vi "GameController.vi"() -> ()   [LabVIEW 2026]
uses:
  <vilib>/Utility/config.llb/Read Key (String).vi
  Instance          15 22Saved   GameController .vi
  <vilib>/Utility/config.llb/Write Key (String).vi
  <vilib>/Instr/_visa.llb/VISA Configure Serial Port (Instr).vi
  <vilib>/Utility/config.llb/NI_LVConfig.lvlib
panel:
  out "Team / Player":string
  out "COM Port":bool
  out "Communication":bool
  in  "Tab Control":T1(tab)
  in  "Final Jeopardy Time":u8=30
  out "Used 7":string
  in  "Final Jeopardy":path
  in  "Question Time":u8=10
  in  "Answer Time":u8=5
  in  "Initialize Moderator Module":bool
  in  "COM Port":refnum<visa-resource-name>
  in  "Point Multiplier":u16(ring) items=["Normal Points", "Double Points"]
  in  "Wrong Sound":path=path "C:/Program Files/BetaBowl/Controller/WrongSound.wav"
  in  "Right Sound":path=path "C:/Program Files/BetaBowl/Controller/RightSound.wav"
  out "Used 6":string
  out "Used 5":string
  out "Used 4":string
  out "Used 3":string
  out "Used 2":string
  out "Used 1":string
  in  "Start Game":bool
  in  "Question Setting":u16(ring) items=["Play & Display Questions", "Display Questions Only"]
  in  "Teams":u16(ring) items=["Two Teams", "Three Teams"]
  in  "Category 6":path
  in  "Category 5":path
  in  "Category 4":path
  in  "Category 3":path
  in  "Category 2":path
  in  "Category 1":path
  in  "Final Jeopardy":bool
  out "GameGUI":bool[][](array[boolean])
  in  "Play/Display Question":bool
  out "Answer":string
  out "Question":string
  in  "TEAM 3":string="0"
  in  "TEAM 2":string="0"
  in  "TEAM 1":string="0"
  in  "WRONG":bool
  in  "RIGHT":bool
  in  "Play/Display":bool
  out "Special Answer":string
  out "Special Question":string
  in  "Team 3 W/R?":bool
  in  "Team 2 W/R?":bool
  in  "Team 1 W/R?":bool
  in  "Dialog Done":bool
  in  "WAGER TEAM 3":string="0"
  in  "WAGER TEAM 2":string="0"
  in  "WAGER TEAM 1":string="0"
  out "Received Message":string
  out "Stats":i32[](array[numeric])
  out "Is Daily Double or Final Jeopardy":bool
  out "Game Started":bool
  out "Timeout":bool
  in  "Start New Question":bool
  out "Com Msgs":string
  out "Daily Double Questions":i32[](array[numeric])
  out "Daily Double Categories":i32[](array[numeric])
  in  "Button Pressed":i32
  in  "Team Pressed":i32
  out "Question":u8
  out "Category":u8
  in  "stop":bool
  # "Category"
  # "Last Used"
  # "1"
  # "2"
  # "3"
  # "4"
  # "5"
  # "6"
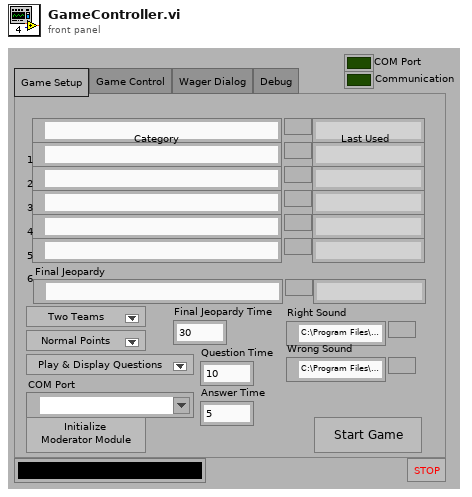
[diagram p1: front panel]
types:
  T1 = enum32{"Game Setup", "Game Control", "Wager Dialog", "Debug"}
  T2 = enum32{"Game Setup", "Game Control", "Wager Dialog"}
  T3 = typedef "NI_LVConfig.lvlib/Config Data RefNum.ctl" = refnum<k1>
  T4 = typedef "Sound Format.ctl" = cluster{"sound quality":enum16{"mono", "stereo"}, "rate":enum16{"11025", "22050", "44100", "8000"}, "bits per sample":enum16{"8 bit", "16 bit"}}
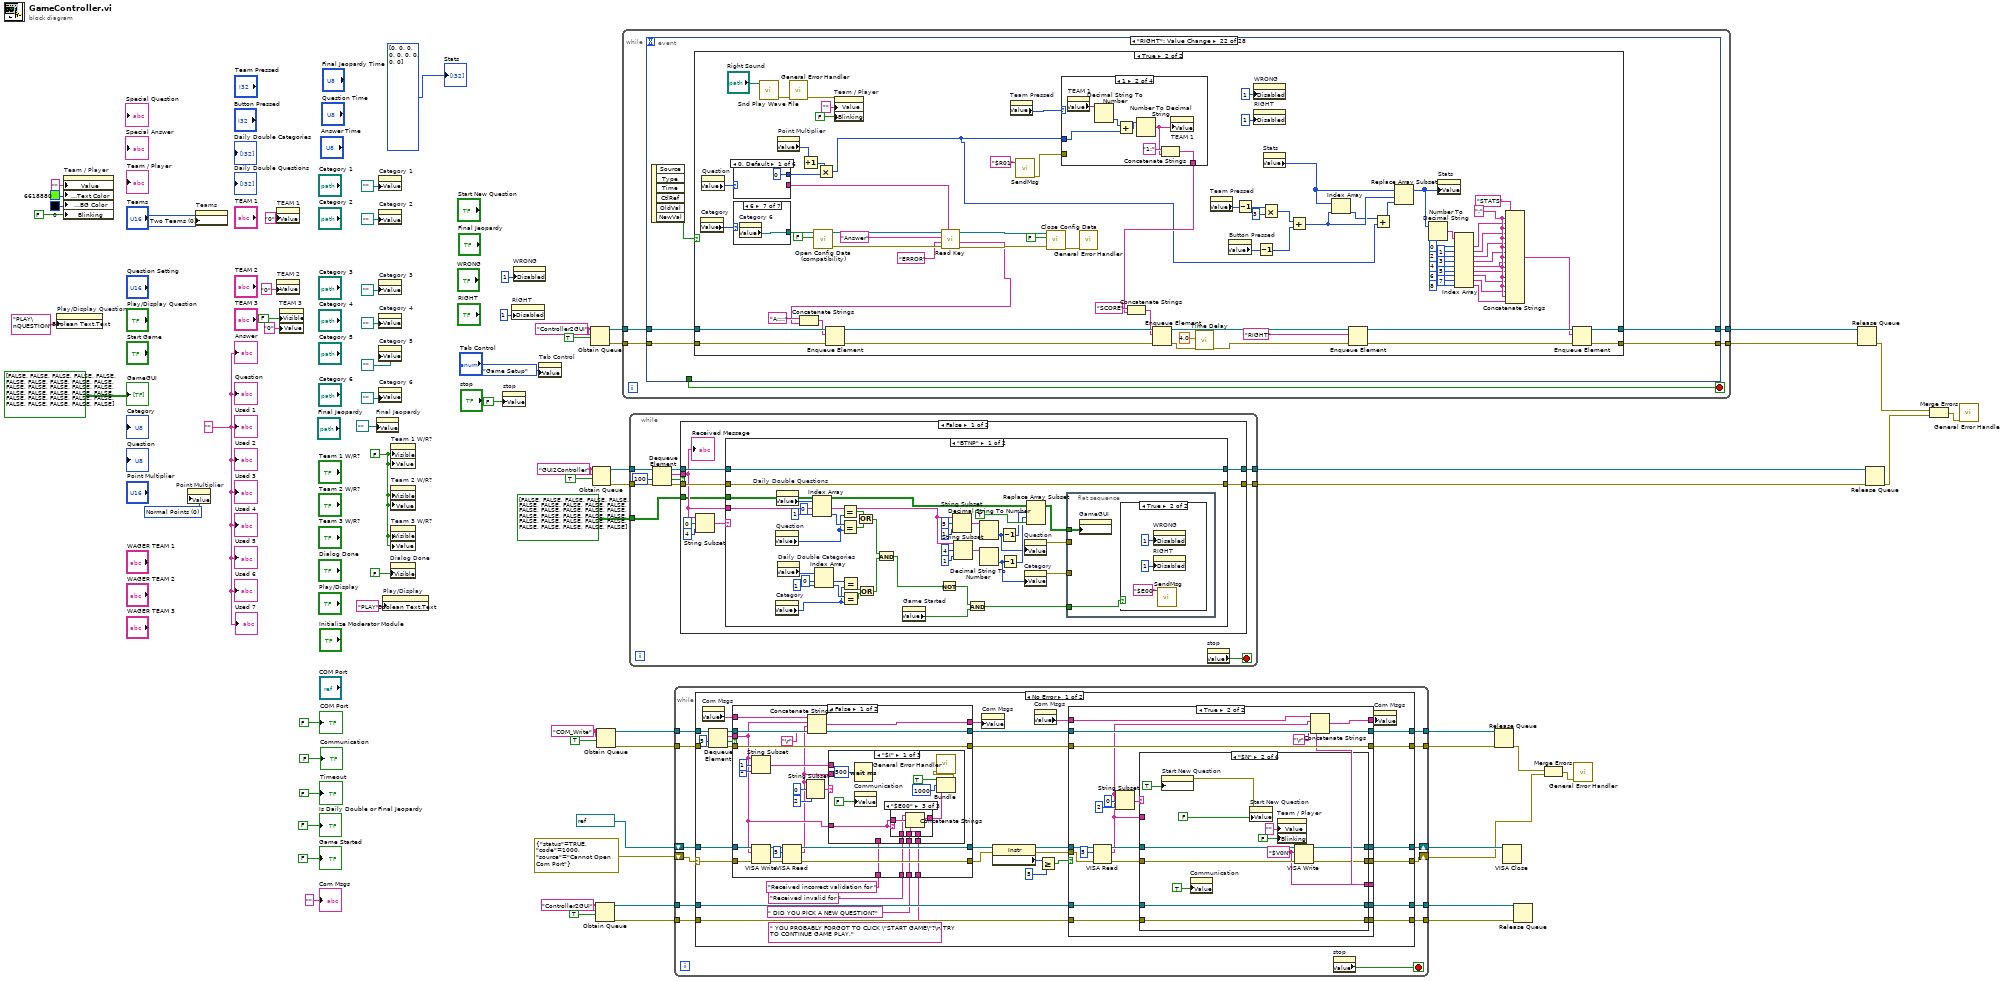
[diagram p0: block diagram]
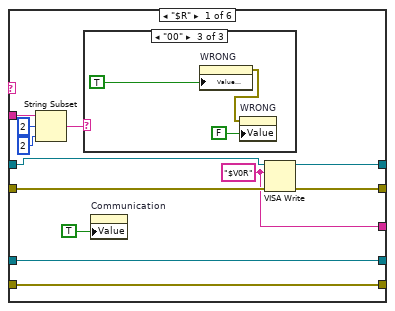
[diagram p3: hidden frame]
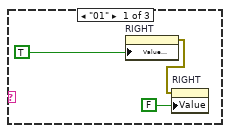
[diagram p4: hidden frame]
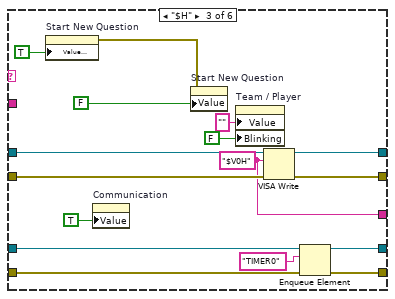
[diagram p6: hidden frame]
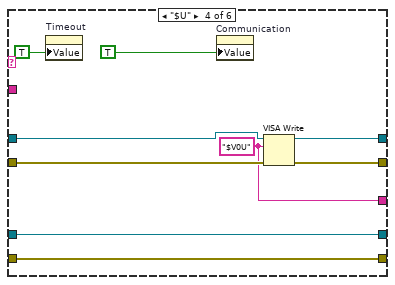
[diagram p7: hidden frame]
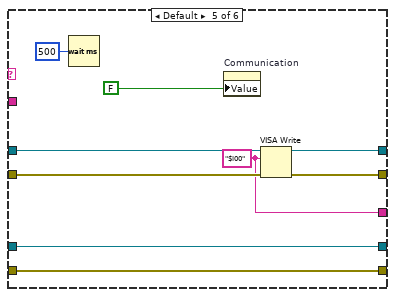
[diagram p8: hidden frame]
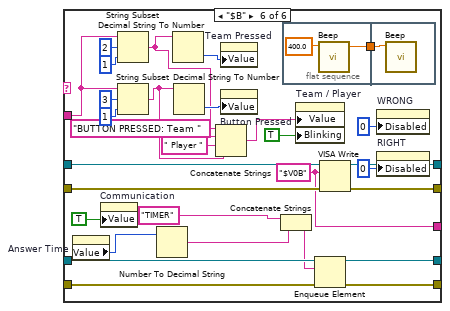
[diagram p9: hidden frame]
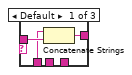
[diagram p10: hidden frame]
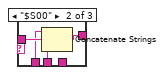
[diagram p11: hidden frame]
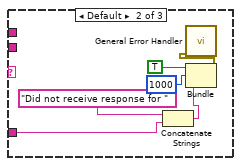
[diagram p12: hidden frame]
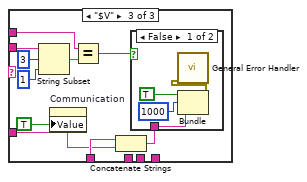
[diagram p13: hidden frame]
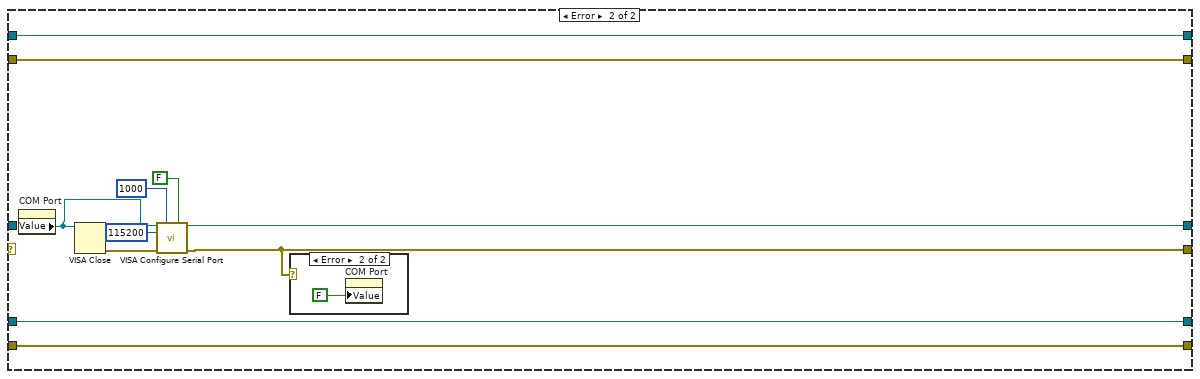
[diagram p16: hidden frame]
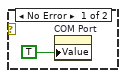
[diagram p17: hidden frame]
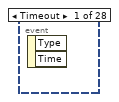
[diagram p18: hidden frame]
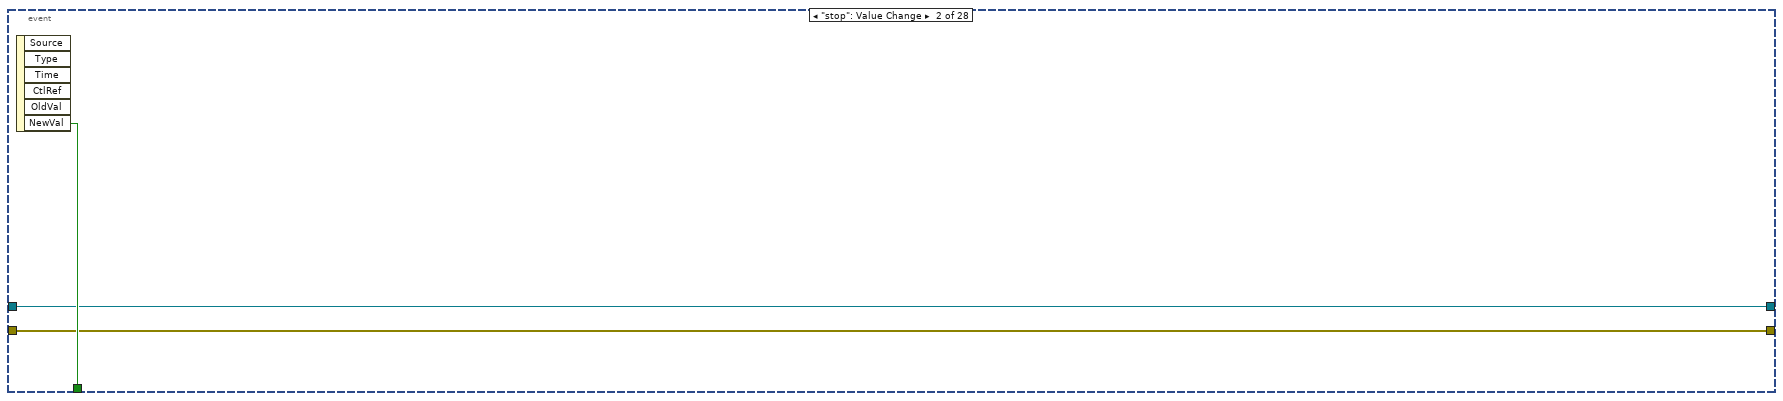
[diagram p19: hidden frame]
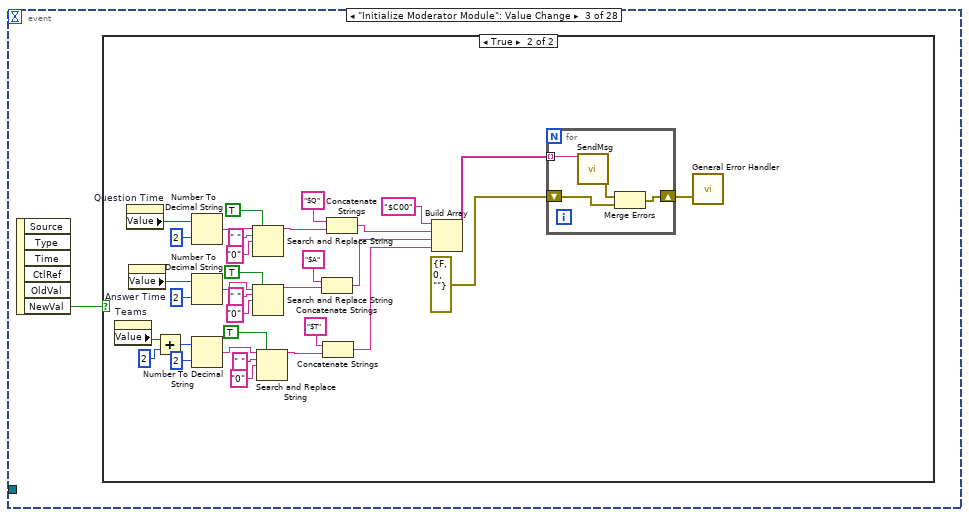
[diagram p20: hidden frame]
diagram:
  w17 = "Controller2GUI" ("name (unnamed)")
  w31 = "COM_Write" ("name (unnamed)")
  w34 = u16 0 items=["Normal Points", "Double Points"] ("Point Multiplier")
  w38 = FALSE ("Visible")
  w4 = "" ("Modified 1")
  w47 = u16 0 items=["Two Teams", "Three Teams"] ("Teams")
  w61 = "Controller2GUI" ("name (unnamed)")
  w68 = "GUI2Controller" ("name (unnamed)")
  n1 = property on="Play/Display Question" class="Bool (strict)"("Boolean Text.Text"="PLAY\nQUESTION") -> ()  [unwired: 2 in, 2 out]
  n2 = property on="Team / Player" class="Str"("Value"="" ("Team / Player"), "Text.Text Colors:Text Color"=u32 6618880, "Text.Text Colors:BG Color"=u32 0, "Blinking"=FALSE) -> ()  [unwired: 2 in, 2 out]
  n3 = property on="Point Multiplier" class="Ring (strict)"("Value"=w34) -> ()  [unwired: 2 in, 2 out]
  n4 = property on="Teams" class="Ring (strict)"("Value (Signaling)"=w47) -> ()  [unwired: 2 in, 2 out]
  n5 = property on="TEAM 1" class="Str"("Value"="0" ("TEAM 1")) -> ()  [unwired: 2 in, 2 out]
  n6 = property on="TEAM 2" class="Str"("Value"="0" ("TEAM 2")) -> ()  [unwired: 2 in, 2 out]
  n7 = property on="TEAM 3" class="Str"("Visible"=FALSE, "Value"="0" ("TEAM 3")) -> ()  [unwired: 2 in, 2 out]
  n8 = property on="Final Jeopardy" class="Path"("Value"=path "" ("Final Jeopardy")) -> ()  [unwired: 2 in, 2 out]
  n9 = property on="Category 1" class="Path"("Value"=path "" ("Category 1")) -> ()  [unwired: 2 in, 2 out]
  n10 = property on="Category 2" class="Path"("Value"=path "" ("Category 2")) -> ()  [unwired: 2 in, 2 out]
  n11 = property on="Category 3" class="Path"("Value"=path "" ("Category 3")) -> ()  [unwired: 2 in, 2 out]
  n12 = property on="Category 4" class="Path"("Value"=path "" ("Category 4")) -> ()  [unwired: 2 in, 2 out]
  n13 = property on="Category 5" class="Path"("Value"=path "" ("Category 5")) -> ()  [unwired: 2 in, 2 out]
  n14 = property on="Category 6" class="Path"("Value"=path "" ("Category 6")) -> ()  [unwired: 2 in, 2 out]
  n15 = property on="Play/Display" class="Bool (strict)"("Boolean Text.Text"="PLAY") -> ()  [unwired: 2 in, 2 out]
  n16 = property on="Dialog Done" class="Bool (strict)"("Visible"=FALSE) -> ()  [unwired: 2 in, 2 out]
  n17 = property on="Team 1 W/R?" class="Bool (strict)"("Visible"=w38, "Value"=w38) -> ()  [unwired: 2 in, 2 out]
  n18 = property on="Team 2 W/R?" class="Bool (strict)"("Visible"=w38, "Value"=w38) -> ()  [unwired: 2 in, 2 out]
  n19 = property on="Team 3 W/R?" class="Bool (strict)"("Visible"=w38, "Value"=w38) -> ()  [unwired: 2 in, 2 out]
  n20 = property on="stop" class="Bool (strict)"("Value"=FALSE ("stop")) -> ()  [unwired: 2 in, 2 out]
  n21 = property on="RIGHT" class="Bool (strict)"("Disabled"=u8 1) -> ()  [unwired: 2 in, 2 out]
  n22 = property on="WRONG" class="Bool (strict)"("Disabled"=u8 1) -> ()  [unwired: 2 in, 2 out]
  n23 = property on="Tab Control" class="TabCtl (strict)"("Value"=T2."Game Setup" ("Tab Control")) -> ()  [unwired: 2 in, 2 out]
  n24 = Obtain Queue(name (unnamed)=w61, element data type=w61, create if not found? (T)=TRUE) -> (queue out=w59:refnum<queue>, error out=w60:errorcluster)  [unwired: 2 in, 1 out]
  n25 = Obtain Queue(name (unnamed)=w68, element data type=w68, create if not found? (T)=TRUE) -> (queue out=w65:refnum<queue>, error out=w66:errorcluster)  [unwired: 2 in, 1 out]
  n26 = Obtain Queue(name (unnamed)=w17, element data type=w17, create if not found? (T)=TRUE) -> (queue out=w15:refnum<queue>, error out=w14:errorcluster)  [unwired: 2 in, 1 out]
  n27 = Obtain Queue(name (unnamed)=w31, element data type=w31, create if not found? (T)=TRUE) -> (queue out=w29:refnum<queue>, error out=w30:errorcluster)  [unwired: 2 in, 1 out]
  n28 = while {
    tunnel: w60 -> [w72]
    tunnel: w59 -> [w71]
    tunnel: [w70] -> w58
    tunnel: [w69] -> w57
    stop <- w73 stop-if-true
    n29 = event shown="[21] \"RIGHT\": Value Change" {
      selector: _ -> [_ _ _ _ _ _ _ _ _ _ _ _ _ _ _ _ _ _ _ _ _ _ _ _ _ _ _ _]
      dyn-events: _ -> [_ _ _ _ _ _ _ _ _ _ _ _ _ _ _ _ _ _ _ _ _ _ _ _ _ _ _ _]
      timeout: _ -> [_ _ _ _ _ _ _ _ _ _ _ _ _ _ _ _ _ _ _ _ _ _ _ _ _ _ _ _]
      tunnel: [_ w76 _ _ _ _ _ _ _ _ _ _ _ _ _ _ _ _ _ _ _ _ _ _ _ _ _ _] -> w73
      tunnel: w72 -> [_ w74 _ w128 w152 w175 w198 w221 w244 w253 w273 w291 w298 w305 w310 w317 w324 w330 _ w417 w438 w454 w578 w711 w762 w866 _ w1124]
      tunnel: w71 -> [_ w75 _ w129 w153 w176 w199 w222 w245 w254 w274 w292 w299 w306 w311 w318 w325 w331 _ w418 w439 w455 w579 w712 w763 w867 _ w1125]
      tunnel: [_ w75 _ w127 w151 w174 w197 w220 w243 w254 w272 w287 w294 w301 w308 w315 w322 w329 _ w416 w437 w453 w577 w710 w761 w865 _ w1123] -> w70
      tunnel: [_ w74 _ w126 w150 w173 w196 w219 w242 w253 w271 w286 w293 w300 w307 w314 w321 w328 _ w415 w436 w452 w576 w709 w760 w864 _ w1122] -> w69
      event Timeout {
        n30 = event-data() -> ()  [unwired: 1 in, 2 out]
      }
      event "stop": Value Change {
        n31 = event-data() -> ("NewVal"=w76:bool)  [unwired: 1 in, 5 out]
      }
      event "Initialize Moderator Module": Value Change {
        n32 = event-data() -> ("NewVal"=w77:bool)  [unwired: 1 in, 5 out]
        n33 = case shown="True" w77 {
          frame False {
          }
          frame True {
            n34 = property on="Teams" class="Ring (strict)"() -> ("Value"=w79:u16)  [unwired: 2 in, 2 out]
            n35 = property on="Question Time" class="DigNum (strict)"() -> ("Value"=w106:u8)  [unwired: 2 in, 2 out]
            n36 = property on="Answer Time" class="DigNum (strict)"() -> ("Value"=w107:u8)  [unwired: 2 in, 2 out]
            n37 = Add(x=w79, y=u16 2) -> (x+y=w80:u16)
            n38 = Number To Decimal String(number=w106, width (-)=i16 2) -> (decimal integer string=w95:string)
            n39 = Number To Decimal String(number=w107, width (-)=i16 2) -> (decimal integer string=w84:string)
            n40 = Number To Decimal String(number=w80, width (-)=i16 2) -> (decimal integer string=w82:string)
            n41 = Search and Replace String(replace all?=TRUE ("replace all? (F)"), input string=w95, search string=" ", replace string="0" ("replace string (\"\")")) -> (result string=w94:string)  [unwired: 4 in, 3 out]
            n42 = Search and Replace String(replace all?=TRUE ("replace all? (F)"), input string=w84, search string=" ", replace string="0" ("replace string (\"\")")) -> (result string=w83:string)  [unwired: 4 in, 3 out]
            n43 = Search and Replace String(replace all?=TRUE ("replace all? (F)"), input string=w82, search string=" ", replace string="0" ("replace string (\"\")")) -> (result string=w81:string)  [unwired: 4 in, 3 out]
            n44 = Concatenate Strings("$A", w83) -> (w100:string)
            n45 = Concatenate Strings("$T", w81) -> (w97:string)
            n46 = Concatenate Strings("$Q", w94) -> (w102:string)
            n47 = Build Array("$C00", w102, w100, w97) -> (w109:string[])
            n48 = for {
              shift-right: [w112] -> w96
              shift-left: errorcluster {"status"=FALSE, "code"=0, "source"=""} ("error in (no error)") -> [w113]
              tunnel: w109 -> [w111] mode=indexing
              n49 = call "SendMsg.vi"("Data"=w111) -> ("error out"=w114:errorcluster)  [unwired: 14 in]
              n50 = Merge Errors(w114, w113) -> (w112:errorcluster)
            }
            n51 = call <vilib>:"General Error Handler.vi"("error in (no error)"=w96) -> ()  [unwired: 10 in, 5 out]
          }
        }
      }
      event "Category 1": Value Change {
        n52 = event-data() -> ("NewVal"=w137:path)  [unwired: 1 in, 5 out]
        n53 = call <vilib>:"Open Config Data (compatibility).vi"("create file if necessary (T)"=FALSE ("create file if necessary? (T)"), "configuration file path"=w137) -> ("error out"=w134:errorcluster, "refnum"=w135:T3)  [unwired: 7 in, 1 out]
        n54 = call-poly <vilib>:"Read Key.vi"("section"="HEADER", "error in (no error)"=w134, "default value"="ERROR" ("key"), "key"="CategoryName", "refnum"=w135) -> ("error out"=w120:errorcluster, "value"=w123:string, "refnum out"=w122:T3)  [unwired: 3 in, 1 out]
        n55 = Concatenate Strings("CAT1:" ("string"), w123) -> (w125:string)
        n56 = call-poly <vilib>:"Read Key.vi"("section"="HEADER", "error in (no error)"=w120, "default value"="ERROR" ("key"), "key"="Used", "refnum"=w122) -> ("error out"=w119:errorcluster, "value"=w115:string, "refnum out"=w121:T3)  [unwired: 3 in, 1 out]
        n57 = property on="Used 1" class="Str"("Value"=w115) -> ()  [unwired: 2 in, 2 out]
        n58 = Enqueue Element(queue=w129, element=w125, error in (no error)=w128) -> (queue out=w127:refnum<queue>, error out=w126:errorcluster)  [unwired: 1 in, 1 out]
        n59 = call <vilib>:"Close Config Data.vi"("error in (no error)"=w119, "write file if changed (T)"=FALSE ("write configuration file? (T)"), "refnum"=w121) -> ()  [unwired: 7 in, 2 out]
      }
      event "Category 2": Value Change {
        n60 = event-data() -> ("NewVal"=w160:path)  [unwired: 1 in, 5 out]
        n61 = call <vilib>:"Open Config Data (compatibility).vi"("create file if necessary (T)"=FALSE ("create file if necessary? (T)"), "configuration file path"=w160) -> ("error out"=w157:errorcluster, "refnum"=w158:T3)  [unwired: 7 in, 1 out]
        n62 = call-poly <vilib>:"Read Key.vi"("section"="HEADER", "error in (no error)"=w157, "default value"="ERROR" ("key"), "key"="CategoryName", "refnum"=w158) -> ("error out"=w139:errorcluster, "value"=w147:string, "refnum out"=w140:T3)  [unwired: 3 in, 1 out]
        n63 = Concatenate Strings("CAT2:" ("string"), w147) -> (w149:string)
        n64 = call-poly <vilib>:"Read Key.vi"("section"="HEADER", "error in (no error)"=w139, "default value"="ERROR" ("key"), "key"="Used", "refnum"=w140) -> ("error out"=w144:errorcluster, "value"=w138:string, "refnum out"=w145:T3)  [unwired: 3 in, 1 out]
        n65 = property on="Used 2" class="Str"("Value"=w138) -> ()  [unwired: 2 in, 2 out]
        n66 = Enqueue Element(queue=w153, element=w149, error in (no error)=w152) -> (queue out=w151:refnum<queue>, error out=w150:errorcluster)  [unwired: 1 in, 1 out]
        n67 = call <vilib>:"Close Config Data.vi"("error in (no error)"=w144, "write file if changed (T)"=FALSE ("write configuration file? (T)"), "refnum"=w145) -> ()  [unwired: 7 in, 2 out]
      }
      event "Category 3": Value Change {
        n68 = event-data() -> ("NewVal"=w183:path)  [unwired: 1 in, 5 out]
        n69 = call <vilib>:"Open Config Data (compatibility).vi"("create file if necessary (T)"=FALSE ("create file if necessary? (T)"), "configuration file path"=w183) -> ("error out"=w180:errorcluster, "refnum"=w181:T3)  [unwired: 7 in, 1 out]
        n70 = call-poly <vilib>:"Read Key.vi"("section"="HEADER", "error in (no error)"=w180, "default value"="ERROR" ("key"), "key"="CategoryName", "refnum"=w181) -> ("error out"=w162:errorcluster, "value"=w170:string, "refnum out"=w163:T3)  [unwired: 3 in, 1 out]
        n71 = Concatenate Strings("CAT3:" ("string"), w170) -> (w172:string)
        n72 = call-poly <vilib>:"Read Key.vi"("section"="HEADER", "error in (no error)"=w162, "default value"="ERROR" ("key"), "key"="Used", "refnum"=w163) -> ("error out"=w166:errorcluster, "value"=w161:string, "refnum out"=w167:T3)  [unwired: 3 in, 1 out]
        n73 = Enqueue Element(queue=w176, element=w172, error in (no error)=w175) -> (queue out=w174:refnum<queue>, error out=w173:errorcluster)  [unwired: 1 in, 1 out]
        n74 = property on="Used 3" class="Str"("Value"=w161) -> ()  [unwired: 2 in, 2 out]
        n75 = call <vilib>:"Close Config Data.vi"("error in (no error)"=w166, "write file if changed (T)"=FALSE ("write configuration file? (T)"), "refnum"=w167) -> ()  [unwired: 7 in, 2 out]
      }
      event "Category 4": Value Change {
        n76 = event-data() -> ("NewVal"=w206:path)  [unwired: 1 in, 5 out]
        n77 = call <vilib>:"Open Config Data (compatibility).vi"("create file if necessary (T)"=FALSE ("create file if necessary? (T)"), "configuration file path"=w206) -> ("error out"=w203:errorcluster, "refnum"=w204:T3)  [unwired: 7 in, 1 out]
        n78 = call-poly <vilib>:"Read Key.vi"("section"="HEADER", "error in (no error)"=w203, "default value"="ERROR" ("key"), "key"="CategoryName", "refnum"=w204) -> ("error out"=w185:errorcluster, "value"=w193:string, "refnum out"=w186:T3)  [unwired: 3 in, 1 out]
        n79 = Concatenate Strings("CAT4:" ("string"), w193) -> (w195:string)
        n80 = call-poly <vilib>:"Read Key.vi"("section"="HEADER", "error in (no error)"=w185, "default value"="ERROR" ("key"), "key"="Used", "refnum"=w186) -> ("error out"=w189:errorcluster, "value"=w184:string, "refnum out"=w190:T3)  [unwired: 3 in, 1 out]
        n81 = Enqueue Element(queue=w199, element=w195, error in (no error)=w198) -> (queue out=w197:refnum<queue>, error out=w196:errorcluster)  [unwired: 1 in, 1 out]
        n82 = property on="Used 4" class="Str"("Value"=w184) -> ()  [unwired: 2 in, 2 out]
        n83 = call <vilib>:"Close Config Data.vi"("error in (no error)"=w189, "write file if changed (T)"=FALSE ("write configuration file? (T)"), "refnum"=w190) -> ()  [unwired: 7 in, 2 out]
      }
      event "Category 5": Value Change {
        n84 = event-data() -> ("NewVal"=w229:path)  [unwired: 1 in, 5 out]
        n85 = call <vilib>:"Open Config Data (compatibility).vi"("create file if necessary (T)"=FALSE ("create file if necessary? (T)"), "configuration file path"=w229) -> ("error out"=w226:errorcluster, "refnum"=w227:T3)  [unwired: 7 in, 1 out]
        n86 = call-poly <vilib>:"Read Key.vi"("section"="HEADER", "error in (no error)"=w226, "default value"="ERROR" ("key"), "key"="CategoryName", "refnum"=w227) -> ("error out"=w208:errorcluster, "value"=w216:string, "refnum out"=w209:T3)  [unwired: 3 in, 1 out]
        n87 = Concatenate Strings("CAT5:" ("string"), w216) -> (w218:string)
        n88 = call-poly <vilib>:"Read Key.vi"("section"="HEADER", "error in (no error)"=w208, "default value"="ERROR" ("key"), "key"="Used", "refnum"=w209) -> ("error out"=w212:errorcluster, "value"=w207:string, "refnum out"=w213:T3)  [unwired: 3 in, 1 out]
        n89 = Enqueue Element(queue=w222, element=w218, error in (no error)=w221) -> (queue out=w220:refnum<queue>, error out=w219:errorcluster)  [unwired: 1 in, 1 out]
        n90 = property on="Used 5" class="Str"("Value"=w207) -> ()  [unwired: 2 in, 2 out]
        n91 = call <vilib>:"Close Config Data.vi"("error in (no error)"=w212, "write file if changed (T)"=FALSE ("write configuration file? (T)"), "refnum"=w213) -> ()  [unwired: 7 in, 2 out]
      }
      event "Category 6": Value Change {
        n92 = event-data() -> ("NewVal"=w252:path)  [unwired: 1 in, 5 out]
        n93 = call <vilib>:"Open Config Data (compatibility).vi"("create file if necessary (T)"=FALSE ("create file if necessary? (T)"), "configuration file path"=w252) -> ("error out"=w249:errorcluster, "refnum"=w250:T3)  [unwired: 7 in, 1 out]
        n94 = call-poly <vilib>:"Read Key.vi"("section"="HEADER", "error in (no error)"=w249, "default value"="ERROR" ("key"), "key"="CategoryName", "refnum"=w250) -> ("error out"=w231:errorcluster, "value"=w239:string, "refnum out"=w232:T3)  [unwired: 3 in, 1 out]
        n95 = Concatenate Strings("CAT6:" ("string"), w239) -> (w241:string)
        n96 = call-poly <vilib>:"Read Key.vi"("section"="HEADER", "error in (no error)"=w231, "default value"="ERROR" ("key"), "key"="Used", "refnum"=w232) -> ("error out"=w235:errorcluster, "value"=w230:string, "refnum out"=w236:T3)  [unwired: 3 in, 1 out]
        n97 = Enqueue Element(queue=w245, element=w241, error in (no error)=w244) -> (queue out=w243:refnum<queue>, error out=w242:errorcluster)  [unwired: 1 in, 1 out]
        n98 = property on="Used 6" class="Str"("Value"=w230) -> ()  [unwired: 2 in, 2 out]
        n99 = call <vilib>:"Close Config Data.vi"("error in (no error)"=w235, "write file if changed (T)"=FALSE ("write configuration file? (T)"), "refnum"=w236) -> ()  [unwired: 7 in, 2 out]
      }
      event "Final Jeopardy": Value Change {
        n100 = event-data() -> ("NewVal"=w270:path)  [unwired: 1 in, 5 out]
        n101 = call <vilib>:"Open Config Data (compatibility).vi"("create file if necessary (T)"=FALSE ("create file if necessary? (T)"), "configuration file path"=w270) -> ("error out"=w267:errorcluster, "refnum"=w268:T3)  [unwired: 7 in, 1 out]
        n102 = call-poly <vilib>:"Read Key.vi"("section"="HEADER", "error in (no error)"=w267, "default value"="ERROR" ("key"), "key"="CategoryName", "refnum"=w268) -> ("error out"=w256:errorcluster, "refnum out"=w257:T3)  [unwired: 3 in, 2 out]
        n103 = call-poly <vilib>:"Read Key.vi"("section"="HEADER", "error in (no error)"=w256, "default value"="ERROR" ("key"), "key"="Used", "refnum"=w257) -> ("error out"=w260:errorcluster, "value"=w255:string, "refnum out"=w261:T3)  [unwired: 3 in, 1 out]
        n104 = property on="Used 7" class="Str"("Value"=w255) -> ()  [unwired: 2 in, 2 out]
        n105 = call <vilib>:"Close Config Data.vi"("error in (no error)"=w260, "write file if changed (T)"=FALSE ("write configuration file? (T)"), "refnum"=w261) -> ()  [unwired: 7 in, 2 out]
      }
      event "Start New Question": Value Change {
        n106 = event-data() -> ("NewVal"=w275:bool)  [unwired: 1 in, 5 out]
        n107 = case shown="True" w275 {
          tunnel: w274 -> [w277 w281]
          tunnel: w273 -> [w276 w280]
          tunnel: [w277 w284] -> w272
          tunnel: [w276 w283] -> w271
          frame False {
          }
          frame True {
            n108 = Enqueue Element(queue=w281, element="TAB::BOARD", error in (no error)=w280) -> (queue out=w278:refnum<queue>, error out=w279:errorcluster)  [unwired: 1 in, 1 out]
            n109 = Enqueue Element(queue=w278, element="UNLOC", error in (no error)=w279) -> (queue out=w284:refnum<queue>, error out=w283:errorcluster)  [unwired: 1 in, 1 out]
          }
        }
      }
      event "TEAM 1": Value Change {
        n110 = event-data() -> ("NewVal"=w289:string)  [unwired: 1 in, 5 out]
        n111 = Concatenate Strings("SCORE1:" ("string"), w289) -> (w288:string)
        n112 = Enqueue Element(queue=w292, element=w288, error in (no error)=w291) -> (queue out=w287:refnum<queue>, error out=w286:errorcluster)  [unwired: 1 in, 1 out]
      }
      event "TEAM 2": Value Change {
        n113 = event-data() -> ("NewVal"=w296:string)  [unwired: 1 in, 5 out]
        n114 = Concatenate Strings("SCORE2:" ("string"), w296) -> (w295:string)
        n115 = Enqueue Element(queue=w299, element=w295, error in (no error)=w298) -> (queue out=w294:refnum<queue>, error out=w293:errorcluster)  [unwired: 1 in, 1 out]
      }
      event "TEAM 3": Value Change {
        n116 = event-data() -> ("NewVal"=w303:string)  [unwired: 1 in, 5 out]
        n117 = Concatenate Strings("SCORE3:" ("string"), w303) -> (w302:string)
        n118 = Enqueue Element(queue=w306, element=w302, error in (no error)=w305) -> (queue out=w301:refnum<queue>, error out=w300:errorcluster)  [unwired: 1 in, 1 out]
      }
      event "WAGER TEAM 1": Value Change {
        n119 = event-data() -> ("NewVal"=w309:string)  [unwired: 1 in, 5 out]
        n120 = Concatenate Strings("WT1::" ("string"), w309) -> (w312:string)
        n121 = Enqueue Element(queue=w311, element=w312, error in (no error)=w310) -> (queue out=w308:refnum<queue>, error out=w307:errorcluster)  [unwired: 1 in, 1 out]
      }
      event "WAGER TEAM 2": Value Change {
        n122 = event-data() -> ("NewVal"=w316:string)  [unwired: 1 in, 5 out]
        n123 = Concatenate Strings("WT2::" ("string"), w316) -> (w319:string)
        n124 = Enqueue Element(queue=w318, element=w319, error in (no error)=w317) -> (queue out=w315:refnum<queue>, error out=w314:errorcluster)  [unwired: 1 in, 1 out]
      }
      event "WAGER TEAM 3": Value Change {
        n125 = event-data() -> ("NewVal"=w323:string)  [unwired: 1 in, 5 out]
        n126 = Concatenate Strings("WT3::" ("string"), w323) -> (w326:string)
        n127 = Enqueue Element(queue=w325, element=w326, error in (no error)=w324) -> (queue out=w322:refnum<queue>, error out=w321:errorcluster)  [unwired: 1 in, 1 out]
      }
      event "Dialog Done": Value Change {
        n128 = event-data() -> ("NewVal"=w332:bool)  [unwired: 1 in, 5 out]
        n129 = case shown="True" w332 {
          tunnel: w331 -> [w333 w336]
          tunnel: w330 -> [w334 w335]
          tunnel: [w333 w360] -> w329
          tunnel: [w334 w359] -> w328
          frame False {
          }
          frame True {
            n130 = property on="Tab Control" class="TabCtl (strict)"("Value"=T2."Game Control" ("Tab Control")) -> (error out=w388:errorcluster)  [unwired: 2 in, 1 out]
            n131 = Enqueue Element(queue=w336, element="TIMER0", error in (no error)=w335) -> (queue out=w337:refnum<queue>, error out=w338:errorcluster)  [unwired: 1 in, 1 out]
            n132 = property on="WAGER TEAM 2" class="Str"() -> ("Value"=w367:string)  [unwired: 2 in, 2 out]
            n133 = property on="WAGER TEAM 3" class="Str"() -> ("Value"=w366:string)  [unwired: 2 in, 2 out]
            n134 = property on="WAGER TEAM 1" class="Str"() -> ("Value"=w368:string)  [unwired: 2 in, 2 out]
            n135 = property on="Dialog Done" class="Bool (strict)"(error in=w388, "Visible"=FALSE) -> ()  [unwired: 1 in, 2 out]
            n136 = Decimal String To Number(string=w368) -> (number=w365:i32)  [unwired: 2 in, 1 out]
            n137 = Decimal String To Number(string=w367) -> (number=w350:i32)  [unwired: 2 in, 1 out]
            n138 = Decimal String To Number(string=w366) -> (number=w347:i32)  [unwired: 2 in, 1 out]
            n139 = Enqueue Element(queue=w337, element="UNLOC", error in (no error)=w338) -> (queue out=w385:refnum<queue>, error out=w384:errorcluster)  [unwired: 1 in, 1 out]
            n140 = property on="TEAM 3" class="Str"() -> ("Value"=w377:string)  [unwired: 2 in, 2 out]
            n141 = property on="TEAM 1" class="Str"() -> ("Value"=w372:string)  [unwired: 2 in, 2 out]
            n142 = property on="TEAM 2" class="Str"() -> ("Value"=w369:string)  [unwired: 2 in, 2 out]
            n143 = Decimal String To Number(string=w377) -> (number=w348:i32)  [unwired: 2 in, 1 out]
            n144 = Decimal String To Number(string=w369) -> (number=w351:i32)  [unwired: 2 in, 1 out]
            n145 = Decimal String To Number(string=w372) -> (number=w373:i32)  [unwired: 2 in, 1 out]
            n146 = property on="Team 2 W/R?" class="Bool (strict)"() -> ("Value"=w345:bool)  [unwired: 2 in, 2 out]
            n147 = property on="Team 1 W/R?" class="Bool (strict)"() -> ("Value"=w352:bool)  [unwired: 2 in, 2 out]
            n148 = property on="Team 3 W/R?" class="Bool (strict)"() -> ("Value"=w344:bool)  [unwired: 2 in, 2 out]
            n149 = Enqueue Element(queue=w385, element="Q::::", error in (no error)=w384) -> (queue out=w381:refnum<queue>, error out=w380:errorcluster)  [unwired: 1 in, 1 out]
            n150 = case shown="False" w352 {
              tunnel: [w405 w408] -> w374
              tunnel: w373 -> [w404 w407]
              tunnel: w365 -> [w403 w406]
              frame True {
                n151 = Subtract(x=w404, y=w403) -> (x-y=w405:i32)
              }
              frame False {
                n152 = Add(x=w407, y=w406) -> (x+y=w408:i32)
              }
            }
            n153 = case shown="False" w345 {
              tunnel: [w399 w402] -> w349
              tunnel: w351 -> [w398 w401]
              tunnel: w350 -> [w397 w400]
              frame True {
                n154 = Subtract(x=w398, y=w397) -> (x-y=w399:i32)
              }
              frame False {
                n155 = Add(x=w401, y=w400) -> (x+y=w402:i32)
              }
            }
            n156 = case shown="False" w344 {
              tunnel: [w393 w396] -> w346
              tunnel: w348 -> [w392 w395]
              tunnel: w347 -> [w391 w394]
              frame True {
                n157 = Subtract(x=w392, y=w391) -> (x-y=w393:i32)
              }
              frame False {
                n158 = Add(x=w395, y=w394) -> (x+y=w396:i32)
              }
            }
            n159 = Enqueue Element(queue=w381, element="A::::", error in (no error)=w380) -> (queue out=w343:refnum<queue>, error out=w341:errorcluster)  [unwired: 1 in, 1 out]
            n160 = Number To Decimal String(number=w349) -> (decimal integer string=w371:string)  [unwired: 1 in]
            n161 = Number To Decimal String(number=w374) -> (decimal integer string=w376:string)  [unwired: 1 in]
            n162 = Number To Decimal String(number=w346) -> (decimal integer string=w379:string)  [unwired: 1 in]
            n163 = Concatenate Strings("SCORE2:" ("string"), w371) -> (w357:string)
            n164 = property on="TEAM 3" class="Str"("Value"=w379) -> (error out=w353:errorcluster)  [unwired: 2 in, 1 out]
            n165 = property on="TEAM 2" class="Str"("Value"=w371) -> (error out=w354:errorcluster)  [unwired: 2 in, 1 out]
            n166 = property on="TEAM 1" class="Str"("Value"=w376) -> (error out=w355:errorcluster)  [unwired: 2 in, 1 out]
            n167 = Concatenate Strings("SCORE1:" ("string"), w376) -> (w358:string)
            n168 = Concatenate Strings("SCORE3:" ("string"), w379) -> (w356:string)
            n169 = Enqueue Element(queue=w343, element="TAB::BOARD", error in (no error)=w341) -> (queue out=w342:refnum<queue>, error out=w340:errorcluster)  [unwired: 1 in, 1 out]
            n170 = Enqueue Element(queue=w342, element=w358, error in (no error)=w340) -> (queue out=w364:refnum<queue>, error out=w363:errorcluster)  [unwired: 1 in, 1 out]
            n171 = Enqueue Element(queue=w364, element=w357, error in (no error)=w363) -> (queue out=w361:refnum<queue>, error out=w362:errorcluster)  [unwired: 1 in, 1 out]
            n172 = Enqueue Element(queue=w361, element=w356, error in (no error)=w362) -> (queue out=w360:refnum<queue>, error out=w359:errorcluster)  [unwired: 1 in, 1 out]
            n173 = flat-sequence {
              tunnel: w355 -> [_]
              tunnel: w354 -> [_]
              tunnel: w353 -> [_]
              frame #0 {
                w409 = FALSE ("Visible")
                n174 = property on="Team 1 W/R?" class="Bool (strict)"("Visible"=w409, "Value"=w409) -> ()  [unwired: 2 in, 2 out]
                n175 = property on="Team 2 W/R?" class="Bool (strict)"("Visible"=w409, "Value"=w409) -> ()  [unwired: 2 in, 2 out]
                n176 = property on="Team 3 W/R?" class="Bool (strict)"("Visible"=w409, "Value"=w409) -> ()  [unwired: 2 in, 2 out]
              }
            }
          }
        }
      }
      event "Question Setting": Value Change {
        n177 = event-data() -> ("NewVal"=w410:u16)  [unwired: 1 in, 5 out]
        n178 = case shown="1" w410 {
          frame 0, Default {
            n179 = property on="Play/Display Question" class="Bool (strict)"("Boolean Text.Text"="PLAY\nQUESTION") -> ()  [unwired: 2 in, 2 out]
            n180 = property on="Play/Display" class="Bool (strict)"("Boolean Text.Text"="PLAY") -> ()  [unwired: 2 in, 2 out]
          }
          frame 1 {
            n181 = property on="Play/Display Question" class="Bool (strict)"("Boolean Text.Text"="DISPLAY\nQUESTION") -> ()  [unwired: 2 in, 2 out]
            n182 = property on="Play/Display" class="Bool (strict)"("Boolean Text.Text"="DISPLAY") -> ()  [unwired: 2 in, 2 out]
          }
        }
      }
      event "Teams": Value Change {
        n183 = event-data() -> ("NewVal"=w419:u16)  [unwired: 1 in, 5 out]
        n184 = case shown="0, Default" w419 {
          tunnel: w418 -> [w425 w432]
          tunnel: w417 -> [w424 w431]
          tunnel: [w422 w429] -> w416
          tunnel: [w421 w428] -> w415
          frame 0, Default {
            n185 = property on="TEAM 3" class="Str"("Visible"=FALSE) -> ()  [unwired: 2 in, 2 out]
            n186 = property on="WAGER TEAM 3" class="Str"("Visible"=FALSE) -> ()  [unwired: 2 in, 2 out]
            n187 = Enqueue Element(queue=w425, element="HIDE3", error in (no error)=w424) -> (queue out=w422:refnum<queue>, error out=w421:errorcluster)  [unwired: 1 in, 1 out]
          }
          frame 1 {
            n188 = property on="TEAM 3" class="Str"("Visible"=TRUE) -> ()  [unwired: 2 in, 2 out]
            n189 = property on="WAGER TEAM 3" class="Str"("Visible"=TRUE) -> ()  [unwired: 2 in, 2 out]
            n190 = Enqueue Element(queue=w432, element="SHOW3", error in (no error)=w431) -> (queue out=w429:refnum<queue>, error out=w428:errorcluster)  [unwired: 1 in, 1 out]
          }
        }
      }
      event "Point Multiplier": Value Change {
        n191 = event-data() -> ("NewVal"=w435:u16)  [unwired: 1 in, 5 out]
        n192 = Increment(x=w435) -> (x+1=w434:u16)
        n193 = case shown="1" w434 {
          tunnel: w439 -> [w441 w445 w450]
          tunnel: w438 -> [w440 w444 w449]
          tunnel: [w441 w443 w448] -> w437
          tunnel: [w440 w442 w447] -> w436
          frame 0, Default {
          }
          frame 1 {
            n194 = Enqueue Element(queue=w445, element="RESET1", error in (no error)=w444) -> (queue out=w443:refnum<queue>, error out=w442:errorcluster)  [unwired: 1 in, 1 out]
          }
          frame 2 {
            n195 = Enqueue Element(queue=w450, element="RESET2", error in (no error)=w449) -> (queue out=w448:refnum<queue>, error out=w447:errorcluster)  [unwired: 1 in, 1 out]
          }
        }
      }
      event "RIGHT": Value Change {
        n196 = event-data() -> ("NewVal"=w456:bool)  [unwired: 1 in, 5 out]
        n197 = case shown="True" w456 {
          tunnel: w455 -> [w458 w536]
          tunnel: w454 -> [w457 w535]
          tunnel: [w458 w462] -> w453
          tunnel: [w457 w461] -> w452
          frame False {
          }
          frame True {
            w475 = ":" ("string")
            n198 = property on="Category" class="DigNum (strict)"() -> ("Value"=w532:u8)  [unwired: 2 in, 2 out]
            n199 = property on="Question" class="DigNum (strict)"() -> ("Value"=w531:u8)  [unwired: 2 in, 2 out]
            n200 = case shown="0, Default" w531 {
              tunnel: [_ "QUESTION1" "QUESTION2" "QUESTION3" "QUESTION4" "QUESTION5"] -> w526
              tunnel: [0 100 200 300 400 500] -> w514
              frame 0, Default {
              }
              frame 1 {
              }
              frame 2 {
              }
              frame 3 {
              }
              frame 4 {
              }
              frame 5 {
              }
            }
            n201 = case shown="6" w532 {
              tunnel: [_ w570 w571 w572 w573 w574 w575] -> w530
              frame 0, Default {
              }
              frame 1 {
                n202 = property on="Category 1" class="Path"() -> ("Value"=w570:path)  [unwired: 2 in, 2 out]
              }
              frame 2 {
                n203 = property on="Category 2" class="Path"() -> ("Value"=w571:path)  [unwired: 2 in, 2 out]
              }
              frame 3 {
                n204 = property on="Category 3" class="Path"() -> ("Value"=w572:path)  [unwired: 2 in, 2 out]
              }
              frame 4 {
                n205 = property on="Category 4" class="Path"() -> ("Value"=w573:path)  [unwired: 2 in, 2 out]
              }
              frame 5 {
                n206 = property on="Category 5" class="Path"() -> ("Value"=w574:path)  [unwired: 2 in, 2 out]
              }
              frame 6 {
                n207 = property on="Category 6" class="Path"() -> ("Value"=w575:path)  [unwired: 2 in, 2 out]
              }
            }
            n208 = call <vilib>:"Snd Play Wave File.vi"("wave file path"="Right Sound") -> ("error out"=w515:errorcluster)  [unwired: 9 in, 1 out]
            n209 = property on="Point Multiplier" class="Ring (strict)"() -> ("Value"=w512:u16)  [unwired: 2 in, 2 out]
            n210 = call <vilib>:"General Error Handler.vi"("error in (no error)"=w515) -> ("error out"=w499:errorcluster)  [unwired: 10 in, 4 out]
            n211 = Increment(x=w512) -> (x+1=w513:u16)
            n212 = call <vilib>:"Open Config Data (compatibility).vi"("create file if necessary (T)"=FALSE ("create file if necessary? (T)"), "configuration file path"=w530) -> ("error out"=w528:errorcluster, "refnum"=w527:T3)  [unwired: 7 in, 1 out]
            n213 = Multiply(x=w513, y=w514) -> (x*y=w486:i32)
            n214 = property on="Team / Player" class="Str"(error in=w499, "Value"="" ("Team / Player"), "Blinking"=FALSE) -> ()  [unwired: 1 in, 2 out]
            n215 = call-poly <vilib>:"Read Key.vi"("section"=w526, "error in (no error)"=w528, "default value"="ERROR" ("key"), "key"="Answer", "refnum"=w527) -> ("error out"=w522:errorcluster, "value"=w517:string, "refnum out"=w523:T3)  [unwired: 3 in, 1 out]
            n216 = Concatenate Strings("A::::" ("string"), w517) -> (w518:string)
            n217 = Enqueue Element(queue=w536, element=w518, error in (no error)=w535) -> (queue out=w511:refnum<queue>, error out=w510:errorcluster)  [unwired: 1 in, 1 out]
            n218 = property on="Team Pressed" class="DigNum (strict)"() -> ("Value"=w502:i32)  [unwired: 2 in, 2 out]
            n219 = call "SendMsg.vi"("Data"="$R01") -> ("error out"=w503:errorcluster)  [unwired: 14 in]
            n220 = call <vilib>:"Close Config Data.vi"("error in (no error)"=w522, "write file if changed (T)"=FALSE ("write configuration file? (T)"), "refnum"=w523) -> ("error out"=w520:errorcluster)  [unwired: 7 in, 1 out]
            n221 = case shown="1" w502 {
              tunnel: w486 -> [_ w542 w550 w557]
              tunnel: [_ w538 w546 w552] -> w505
              tunnel: w503 -> [_ _ _ _]
              frame 0, Default {
              }
              frame 1 {
                n222 = property on="TEAM 1" class="Str"() -> ("Value"=w544:string)  [unwired: 2 in, 2 out]
                n223 = Decimal String To Number(string=w544) -> (number=w543:i32)  [unwired: 2 in, 1 out]
                n224 = Add(x=w543, y=w542) -> (x+y=w541:i32)
                n225 = Number To Decimal String(number=w541) -> (decimal integer string=w539:string)  [unwired: 1 in]
                n226 = Concatenate Strings("1:" ("string"), w539) -> (w538:string)
                n227 = property on="TEAM 1" class="Str"("Value"=w539) -> ()  [unwired: 2 in, 2 out]
              }
              frame 2 {
                n228 = property on="TEAM 2" class="Str"() -> ("Value"=w548:string)  [unwired: 2 in, 2 out]
                n229 = Decimal String To Number(string=w548) -> (number=w551:i32)  [unwired: 2 in, 1 out]
                n230 = Add(x=w551, y=w550) -> (x+y=w549:i32)
                n231 = Number To Decimal String(number=w549) -> (decimal integer string=w545:string)  [unwired: 1 in]
                n232 = Concatenate Strings("2:" ("string"), w545) -> (w546:string)
                n233 = property on="TEAM 2" class="Str"("Value"=w545) -> ()  [unwired: 2 in, 2 out]
              }
              frame 3 {
                n234 = property on="TEAM 3" class="Str"() -> ("Value"=w555:string)  [unwired: 2 in, 2 out]
                n235 = Decimal String To Number(string=w555) -> (number=w558:i32)  [unwired: 2 in, 1 out]
                n236 = Add(x=w558, y=w557) -> (x+y=w556:i32)
                n237 = Number To Decimal String(number=w556) -> (decimal integer string=w553:string)  [unwired: 1 in]
                n238 = Concatenate Strings("3:" ("string"), w553) -> (w552:string)
                n239 = property on="TEAM 3" class="Str"("Value"=w553) -> ()  [unwired: 2 in, 2 out]
              }
            }
            n240 = call <vilib>:"General Error Handler.vi"("error in (no error)"=w520) -> ()  [unwired: 10 in, 5 out]
            n241 = Concatenate Strings("SCORE" ("string"), w505) -> (w507:string)
            n242 = Enqueue Element(queue=w511, element=w507, error in (no error)=w510) -> (queue out=w508:refnum<queue>, error out=w509:errorcluster)  [unwired: 1 in, 1 out]
            n243 = call "Time Delay"("error in (no error)"=w509, "Delay Time (s)"=4.0) -> ("error out"=w534:errorcluster)  [unwired: 9 in]
            n244 = property on="Team Pressed" class="DigNum (strict)"() -> ("Value"=w496:i32)  [unwired: 2 in, 2 out]
            n245 = property on="Button Pressed" class="DigNum (strict)"() -> ("Value"=w492:i32)  [unwired: 2 in, 2 out]
            n246 = Decrement(x=w496) -> (x-1=w495:i32)
            n247 = property on="WRONG" class="Bool (strict)"("Disabled"=u8 1) -> ()  [unwired: 2 in, 2 out]
            n248 = property on="RIGHT" class="Bool (strict)"("Disabled"=u8 1) -> ()  [unwired: 2 in, 2 out]
            n249 = Decrement(x=w492) -> (x-1=w491:i32)
            n250 = Multiply(x=w495, y=3) -> (x*y=w493:i32)
            n251 = property on="Stats" class="Arr (strict)"() -> ("Value"=w490:i32[])  [unwired: 2 in, 2 out]
            n252 = Add(x=w493, y=w491) -> (x+y=w489:i32)
            n253 = Index Array(array=w490, index=w489) -> (element=w488:i32)
            n254 = Enqueue Element(queue=w508, element="RIGHT", error in (no error)=w534) -> (queue out=w464:refnum<queue>, error out=w463:errorcluster)  [unwired: 1 in, 1 out]
            n255 = Add(x=w488, y=w486) -> (x+y=w487:i32)
            n256 = Replace Array Subset(array=w490, new element=w487, index=w489) -> (w465:i32[])
            n257 = Number To Decimal String(number=w465) -> (decimal integer string=w485:string[])  [unwired: 1 in]
            n258 = property on="Stats" class="Arr (strict)"("Value"=w465) -> ()  [unwired: 2 in, 2 out]
            n259 = Index Array(array=w485, index #1=0 ("index"), index #2=1 ("index"), index #3=2 ("index"), index #4=3 ("index"), index #5=4 ("index"), index #6=5 ("index"), index #7=6 ("index"), index #8=7 ("index"), index #9=8 ("index")) -> (element #1=w474:string, element #2=w473:string, element #3=w472:string, element #4=w471:string, element #5=w466:string, element #6=w467:string, element #7=w468:string, element #8=w469:string, element #9=w470:string)
            n260 = Concatenate Strings("STATS" ("string"), w475, w474, w475, w473, w475, w472, w475, w471, w475, w466, w475, w467, w475, w468, w475, w469, w475, w470) -> (w460:string)
            n261 = Enqueue Element(queue=w464, element=w460, error in (no error)=w463) -> (queue out=w462:refnum<queue>, error out=w461:errorcluster)  [unwired: 1 in, 1 out]
          }
        }
      }
      event "WRONG": Value Change {
        n262 = event-data() -> ("NewVal"=w580:bool)  [unwired: 1 in, 5 out]
        n263 = case shown="True" w580 {
          tunnel: w579 -> [w582 w654]
          tunnel: w578 -> [w581 w653]
          tunnel: [w582 w585] -> w577
          tunnel: [w581 w584] -> w576
          frame False {
          }
          frame True {
            w598 = ":" ("string")
            n264 = property on="Category" class="DigNum (strict)"() -> ("Value"=w668:u8)  [unwired: 2 in, 2 out]
            n265 = property on="Question" class="DigNum (strict)"() -> ("Value"=w651:u8)  [unwired: 2 in, 2 out]
            n266 = case shown="0, Default" w651 {
              tunnel: [_ "QUESTION1" "QUESTION2" "QUESTION3" "QUESTION4" "QUESTION5"] -> w650
              tunnel: [0 100 200 300 400 500] -> w647
              frame 0, Default {
              }
              frame 1 {
              }
              frame 2 {
              }
              frame 3 {
              }
              frame 4 {
              }
              frame 5 {
              }
            }
            n267 = case shown="6" w668 {
              tunnel: [_ w703 w704 w705 w706 w707 w708] -> w667
              frame 0, Default {
              }
              frame 1 {
                n268 = property on="Category 1" class="Path"() -> ("Value"=w703:path)  [unwired: 2 in, 2 out]
              }
              frame 2 {
                n269 = property on="Category 2" class="Path"() -> ("Value"=w704:path)  [unwired: 2 in, 2 out]
              }
              frame 3 {
                n270 = property on="Category 3" class="Path"() -> ("Value"=w705:path)  [unwired: 2 in, 2 out]
              }
              frame 4 {
                n271 = property on="Category 4" class="Path"() -> ("Value"=w706:path)  [unwired: 2 in, 2 out]
              }
              frame 5 {
                n272 = property on="Category 5" class="Path"() -> ("Value"=w707:path)  [unwired: 2 in, 2 out]
              }
              frame 6 {
                n273 = property on="Category 6" class="Path"() -> ("Value"=w708:path)  [unwired: 2 in, 2 out]
              }
            }
            n274 = call <vilib>:"Snd Play Wave File.vi"("wave file path"="Wrong Sound") -> ("error out"=w655:errorcluster)  [unwired: 9 in, 1 out]
            n275 = call <vilib>:"General Error Handler.vi"("error in (no error)"=w655) -> ("error out"=w623:errorcluster)  [unwired: 10 in, 4 out]
            n276 = property on="Point Multiplier" class="Ring (strict)"() -> ("Value"=w648:u16)  [unwired: 2 in, 2 out]
            n277 = Concatenate Strings("A::::" ("string"), "" ("string")) -> (w656:string)
            n278 = Increment(x=w648) -> (x+1=w649:u16)
            n279 = call <vilib>:"Open Config Data (compatibility).vi"("create file if necessary (T)"=FALSE ("create file if necessary? (T)"), "configuration file path"=w667) -> ("error out"=w665:errorcluster, "refnum"=w664:T3)  [unwired: 7 in, 1 out]
            n280 = Multiply(x=w649, y=w647) -> (x*y=w610:i32)
            n281 = Enqueue Element(queue=w654, element=w656, error in (no error)=w653) -> (queue out=w632:refnum<queue>, error out=w631:errorcluster)  [unwired: 1 in, 1 out]
            n282 = property on="Question" class="Str"() -> ("Value"=w629:string)  [unwired: 2 in, 2 out]
            n283 = property on="Team / Player" class="Str"(error in=w623, "Value"="" ("Team / Player"), "Blinking"=FALSE) -> ()  [unwired: 1 in, 2 out]
            n284 = Concatenate Strings("Q::::" ("string"), w629) -> (w628:string)
            n285 = Enqueue Element(queue=w632, element=w628, error in (no error)=w631) -> (queue out=w627:refnum<queue>, error out=w626:errorcluster)  [unwired: 1 in, 1 out]
            n286 = property on="Team Pressed" class="DigNum (strict)"() -> ("Value"=w639:i32)  [unwired: 2 in, 2 out]
            n287 = call "SendMsg.vi"("Data"="$R00") -> ("error out"=w640:errorcluster)  [unwired: 14 in]
            n288 = call-poly <vilib>:"Read Key.vi"("section"=w650, "error in (no error)"=w665, "default value"="ERROR" ("key"), "key"="Answer", "refnum"=w664) -> ("error out"=w660:errorcluster, "refnum out"=w661:T3)  [unwired: 3 in, 2 out]
            n289 = case shown="3" w639 {
              tunnel: w610 -> [_ w675 w683 w690]
              tunnel: [_ w671 w679 w685] -> w642
              tunnel: w640 -> [_ _ _ _]
              frame 0, Default {
              }
              frame 1 {
                n290 = property on="TEAM 1" class="Str"() -> ("Value"=w677:string)  [unwired: 2 in, 2 out]
                n291 = Decimal String To Number(string=w677) -> (number=w676:i32)  [unwired: 2 in, 1 out]
                n292 = Subtract(x=w676, y=w675) -> (x-y=w674:i32)
                n293 = Number To Decimal String(number=w674) -> (decimal integer string=w672:string)  [unwired: 1 in]
                n294 = Concatenate Strings("1:" ("string"), w672) -> (w671:string)
                n295 = property on="TEAM 1" class="Str"("Value"=w672) -> ()  [unwired: 2 in, 2 out]
              }
              frame 2 {
                n296 = property on="TEAM 2" class="Str"() -> ("Value"=w681:string)  [unwired: 2 in, 2 out]
                n297 = Decimal String To Number(string=w681) -> (number=w684:i32)  [unwired: 2 in, 1 out]
                n298 = Subtract(x=w684, y=w683) -> (x-y=w682:i32)
                n299 = Number To Decimal String(number=w682) -> (decimal integer string=w678:string)  [unwired: 1 in]
                n300 = Concatenate Strings("2:" ("string"), w678) -> (w679:string)
                n301 = property on="TEAM 2" class="Str"("Value"=w678) -> ()  [unwired: 2 in, 2 out]
              }
              frame 3 {
                n302 = property on="TEAM 3" class="Str"() -> ("Value"=w688:string)  [unwired: 2 in, 2 out]
                n303 = Decimal String To Number(string=w688) -> (number=w691:i32)  [unwired: 2 in, 1 out]
                n304 = Subtract(x=w691, y=w690) -> (x-y=w689:i32)
                n305 = Number To Decimal String(number=w689) -> (decimal integer string=w686:string)  [unwired: 1 in]
                n306 = Concatenate Strings("3:" ("string"), w686) -> (w685:string)
                n307 = property on="TEAM 3" class="Str"("Value"=w686) -> ()  [unwired: 2 in, 2 out]
              }
            }
            n308 = call <vilib>:"Close Config Data.vi"("error in (no error)"=w660, "write file if changed (T)"=FALSE ("write configuration file? (T)"), "refnum"=w661) -> ("error out"=w658:errorcluster)  [unwired: 7 in, 1 out]
            n309 = call <vilib>:"General Error Handler.vi"("error in (no error)"=w658) -> ()  [unwired: 10 in, 5 out]
            n310 = Enqueue Element(queue=w627, element="WRONG", error in (no error)=w626) -> (queue out=w646:refnum<queue>, error out=w645:errorcluster)  [unwired: 1 in, 1 out]
            n311 = Concatenate Strings("SCORE" ("element"), w642) -> (w643:string)
            n312 = property on="Question Time" class="DigNum (strict)"() -> ("Value"=w633:u8)  [unwired: 2 in, 2 out]
            n313 = property on="Team Pressed" class="DigNum (strict)"() -> ("Value"=w620:i32)  [unwired: 2 in, 2 out]
            n314 = Enqueue Element(queue=w646, element=w643, error in (no error)=w645) -> (queue out=w636:refnum<queue>, error out=w635:errorcluster)  [unwired: 1 in, 1 out]
            n315 = property on="WRONG" class="Bool (strict)"("Disabled"=u8 1) -> ()  [unwired: 2 in, 2 out]
            n316 = property on="RIGHT" class="Bool (strict)"("Disabled"=u8 1) -> ()  [unwired: 2 in, 2 out]
            n317 = property on="Button Pressed" class="DigNum (strict)"() -> ("Value"=w616:i32)  [unwired: 2 in, 2 out]
            n318 = Decrement(x=w620) -> (x-1=w619:i32)
            n319 = Number To Decimal String(number=w633) -> (decimal integer string=w637:string)  [unwired: 1 in]
            n320 = Decrement(x=w616) -> (x-1=w615:i32)
            n321 = Multiply(x=w619, y=3) -> (x*y=w617:i32)
            n322 = property on="Stats" class="Arr (strict)"() -> ("Value"=w614:i32[])  [unwired: 2 in, 2 out]
            n323 = Concatenate Strings("TIMER" ("string"), w637) -> (w634:string)
            n324 = Enqueue Element(queue=w636, element=w634, error in (no error)=w635) -> (queue out=w587:refnum<queue>, error out=w586:errorcluster)  [unwired: 1 in, 1 out]
            n325 = Add(x=w617, y=w615) -> (x+y=w613:i32)
            n326 = Index Array(array=w614, index=w613) -> (element=w612:i32)
            n327 = Subtract(x=w612, y=w610) -> (x-y=w611:i32)
            n328 = Replace Array Subset(array=w614, new element=w611, index=w613) -> (w609:i32[])
            n329 = Number To Decimal String(number=w609) -> (decimal integer string=w608:string[])  [unwired: 1 in]
            n330 = property on="Stats" class="Arr (strict)"("Value"=w609) -> ()  [unwired: 2 in, 2 out]
            n331 = Index Array(array=w608, index #1=0 ("index"), index #2=1 ("index"), index #3=2 ("index"), index #4=3 ("index"), index #5=4 ("index"), index #6=5 ("index"), index #7=6 ("index"), index #8=7 ("index"), index #9=8 ("index")) -> (element #1=w597:string, element #2=w596:string, element #3=w595:string, element #4=w594:string, element #5=w589:string, element #6=w590:string, element #7=w591:string, element #8=w592:string, element #9=w593:string)
            n332 = Concatenate Strings("STATS" ("string"), w598, w597, w598, w596, w598, w595, w598, w594, w598, w589, w598, w590, w598, w591, w598, w592, w598, w593) -> (w583:string)
            n333 = Enqueue Element(queue=w587, element=w583, error in (no error)=w586) -> (queue out=w585:refnum<queue>, error out=w584:errorcluster)  [unwired: 1 in, 1 out]
          }
        }
      }
      event "Start Game": Value Change {
        n334 = event-data() -> ("NewVal"=w713:bool)  [unwired: 1 in, 5 out]
        n335 = case shown="True" w713 {
          tunnel: w712 -> [w715 w727]
          tunnel: w711 -> [w714 w726]
          tunnel: [w715 w720] -> w710
          tunnel: [w714 w719] -> w709
          frame False {
          }
          frame True {
            n336 = property on="Point Multiplier" class="Ring (strict)"() -> ("Value"=w725:u16)  [unwired: 2 in, 2 out]
            n337 = while {
              stop <- w728 stop-if-true
              n338 = Random Number (0-1)() -> (number: 0 to 1=w756:dbl)
              n339 = Random Number (0-1)() -> (number: 0 to 1=w751:dbl)
              n340 = Random Number (0-1)() -> (number: 0 to 1=w750:dbl)
              n341 = Random Number (0-1)() -> (number: 0 to 1=w745:dbl)
              n342 = Multiply(x=w756, y=6.0) -> (x*y=w742:dbl)
              n343 = Multiply(x=w751, y=6.0) -> (x*y=w740:dbl)
              n344 = Multiply(x=w750, y=5.0) -> (x*y=w739:dbl)
              n345 = Multiply(x=w745, y=5.0) -> (x*y=w738:dbl)
              n346 = Round Toward -Infinity(1:w742) -> (0:w741:dbl)
              n347 = Round Toward -Infinity(1:w739) -> (0:w736:dbl)
              n348 = Round Toward -Infinity(1:w740) -> (0:w735:dbl)
              n349 = Round Toward -Infinity(1:w738) -> (0:w737:dbl)
              n350 = To Long Integer(number=w741) -> (32bit integer=w754:i32)
              n351 = To Long Integer(number=w735) -> (32bit integer=w753:i32)
              n352 = To Long Integer(number=w736) -> (32bit integer=w748:i32)
              n353 = To Long Integer(number=w737) -> (32bit integer=w747:i32)
              n354 = Increment(x=w754) -> (x+1=w734:i32)
              n355 = Increment(x=w753) -> (x+1=w733:i32)
              n356 = Increment(x=w748) -> (x+1=w732:i32)
              n357 = Increment(x=w747) -> (x+1=w731:i32)
              n358 = Not Equal?(x=w734, y=w733) -> (x != y?=w729:bool)
              n359 = Not Equal?(x=w732, y=w731) -> (x != y?=w730:bool)
              n360 = Build Array(w732, w731) -> (w743:i32[])
              n361 = Build Array(w734, w733) -> (w744:i32[])
              n362 = Or(x=w729, y=w730) -> (x .or. y?=w728:bool)
              n363 = property on="Daily Double Questions" class="Arr (strict)"("Value"=w743) -> ()  [unwired: 2 in, 2 out]
              n364 = property on="Daily Double Categories" class="Arr (strict)"("Value"=w744) -> ()  [unwired: 2 in, 2 out]
            }
            n365 = Increment(x=w725) -> (x+1=w724:u16)
            n366 = case shown="0, Default" w724 {
              tunnel: ["" ("element") "RESET1" ("element") "RESET2" ("element")] -> w723
              frame 0, Default {
              }
              frame 1 {
              }
              frame 2 {
              }
            }
            n367 = property on="Tab Control" class="TabCtl (strict)"("Value"=T2."Game Control" ("Tab Control")) -> ()  [unwired: 2 in, 2 out]
            n368 = Enqueue Element(queue=w727, element=w723, error in (no error)=w726) -> (queue out=w722:refnum<queue>, error out=w721:errorcluster)  [unwired: 1 in, 1 out]
            n369 = property on="Game Started" class="Bool (strict)"("Value"=TRUE ("Game Started")) -> ()  [unwired: 2 in, 2 out]
            n370 = Enqueue Element(queue=w722, element="UNLOC", error in (no error)=w721) -> (queue out=w720:refnum<queue>, error out=w719:errorcluster)  [unwired: 1 in, 1 out]
          }
        }
      }
      event "GameGUI": Value Change {
        n371 = event-data() -> ()  [unwired: 1 in, 6 out]
        n372 = property on="Question" class="DigNum (strict)"() -> ("Value"=w768:u8)  [unwired: 2 in, 2 out]
        n373 = property on="Category" class="DigNum (strict)"() -> ("Value"=w767:u8)  [unwired: 2 in, 2 out]
        n374 = property on="Daily Double Questions" class="Arr (strict)"() -> ("Value"=w777:i32[])  [unwired: 2 in, 2 out]
        n375 = property on="Daily Double Categories" class="Arr (strict)"() -> ("Value"=w769:i32[])  [unwired: 2 in, 2 out]
        n376 = Index Array(array=w777, index #1=0 ("index"), index #2=1 ("index")) -> (element #1=w779:i32, element #2=w780:i32)
        n377 = Index Array(array=w769, index #1=0 ("index"), index #2=1 ("index")) -> (element #1=w772:i32, element #2=w773:i32)
        n378 = Equal?(x=w779, y=w768) -> (x = y?=w781:bool)
        n379 = Equal?(x=w780, y=w768) -> (x = y?=w782:bool)
        n380 = Equal?(x=w772, y=w767) -> (x = y?=w774:bool)
        n381 = Equal?(x=w773, y=w767) -> (x = y?=w775:bool)
        n382 = Or(x=w781, y=w782) -> (x .or. y?=w766:bool)
        n383 = Or(x=w774, y=w775) -> (x .or. y?=w765:bool)
        n384 = And(x=w766, y=w765) -> (x .and. y?=w764:bool)
        n385 = case shown="True" w764 {
          tunnel: w767 -> [w800 w851]
          tunnel: w768 -> [w799 w850]
          tunnel: w763 -> [_ w835]
          tunnel: w762 -> [_ w834]
          tunnel: [_ w820] -> w761
          tunnel: [_ w819] -> w760
          frame False {
            n386 = case shown="6" w799 {
              tunnel: [_ "QUESTION1" "QUESTION2" "QUESTION3" "QUESTION4" "QUESTION5" "QUESTION6"] -> w787
              frame 0, Default {
              }
              frame 1 {
              }
              frame 2 {
              }
              frame 3 {
              }
              frame 4 {
              }
              frame 5 {
              }
              frame 6 {
              }
            }
            n387 = case shown="6" w800 {
              tunnel: [_ w807 w808 w809 w810 w811 w812] -> w798
              frame 0, Default {
              }
              frame 1 {
                n388 = property on="Category 1" class="Path"() -> ("Value"=w807:path)  [unwired: 2 in, 2 out]
              }
              frame 2 {
                n389 = property on="Category 2" class="Path"() -> ("Value"=w808:path)  [unwired: 2 in, 2 out]
              }
              frame 3 {
                n390 = property on="Category 3" class="Path"() -> ("Value"=w809:path)  [unwired: 2 in, 2 out]
              }
              frame 4 {
                n391 = property on="Category 4" class="Path"() -> ("Value"=w810:path)  [unwired: 2 in, 2 out]
              }
              frame 5 {
                n392 = property on="Category 5" class="Path"() -> ("Value"=w811:path)  [unwired: 2 in, 2 out]
              }
              frame 6 {
                n393 = property on="Category 6" class="Path"() -> ("Value"=w812:path)  [unwired: 2 in, 2 out]
              }
            }
            n394 = call <vilib>:"Open Config Data (compatibility).vi"("create file if necessary (T)"=FALSE ("create file if necessary? (T)"), "configuration file path"=w798) -> ("error out"=w794:errorcluster, "refnum"=w796:T3)  [unwired: 7 in, 1 out]
            n395 = call-poly <vilib>:"Read Key.vi"("section"=w787, "error in (no error)"=w794, "default value"="ERROR" ("key"), "key"="Question", "refnum"=w796) -> ("error out"=w790:errorcluster, "value"=w783:string, "refnum out"=w791:T3)  [unwired: 3 in, 1 out]
            n396 = property on="Question" class="Str"("Value"=w783) -> ()  [unwired: 2 in, 2 out]
            n397 = call-poly <vilib>:"Read Key.vi"("section"=w787, "error in (no error)"=w790, "default value"="ERROR" ("key"), "key"="Answer", "refnum"=w791) -> ("error out"=w789:errorcluster, "value"=w784:string, "refnum out"=w788:T3)  [unwired: 3 in, 1 out]
            n398 = property on="Answer" class="Str"("Value"=w784) -> ()  [unwired: 2 in, 2 out]
            n399 = call <vilib>:"Close Config Data.vi"("error in (no error)"=w789, "refnum"=w788) -> ("error out"=w792:errorcluster)  [unwired: 8 in, 1 out]
            n400 = property on="Special Answer" class="Str"("Value"=w784) -> ()  [unwired: 2 in, 2 out]
            n401 = property on="Special Question" class="Str"("Value"=w783) -> ()  [unwired: 2 in, 2 out]
            n402 = call <vilib>:"General Error Handler.vi"("error in (no error)"=w792) -> ()  [unwired: 10 in, 5 out]
          }
          frame True {
            w817 = "0" ("WAGER TEAM 1")
            (unwired) 1 ("Mode")
            n403 = case shown="6" w850 {
              tunnel: [_ "QUESTION1" "QUESTION2" "QUESTION3" "QUESTION4" "QUESTION5" "QUESTION6"] -> w838
              frame 0, Default {
              }
              frame 1 {
              }
              frame 2 {
              }
              frame 3 {
              }
              frame 4 {
              }
              frame 5 {
              }
              frame 6 {
              }
            }
            n404 = case shown="6" w851 {
              tunnel: [_ w858 w859 w860 w861 w862 w863] -> w849
              frame 0, Default {
              }
              frame 1 {
                n405 = property on="Category 1" class="Path"() -> ("Value"=w858:path)  [unwired: 2 in, 2 out]
              }
              frame 2 {
                n406 = property on="Category 2" class="Path"() -> ("Value"=w859:path)  [unwired: 2 in, 2 out]
              }
              frame 3 {
                n407 = property on="Category 3" class="Path"() -> ("Value"=w860:path)  [unwired: 2 in, 2 out]
              }
              frame 4 {
                n408 = property on="Category 4" class="Path"() -> ("Value"=w861:path)  [unwired: 2 in, 2 out]
              }
              frame 5 {
                n409 = property on="Category 5" class="Path"() -> ("Value"=w862:path)  [unwired: 2 in, 2 out]
              }
              frame 6 {
                n410 = property on="Category 6" class="Path"() -> ("Value"=w863:path)  [unwired: 2 in, 2 out]
              }
            }
            n411 = property on="Tab Control" class="TabCtl (strict)"("Value"=T2."Wager Dialog" ("Tab Control")) -> ()  [unwired: 2 in, 2 out]
            n412 = property on="Dialog Done" class="Bool (strict)"("Visible"=FALSE) -> ()  [unwired: 2 in, 2 out]
            n413 = Enqueue Element(queue=w835, element="DIAL:DAILY DOUBLE", error in (no error)=w834) -> (queue out=w832:refnum<queue>, error out=w831:errorcluster)  [unwired: 1 in, 1 out]
            n414 = property on="WAGER TEAM 1" class="Str"("Value"=w817) -> ()  [unwired: 2 in, 2 out]
            n415 = property on="WAGER TEAM 2" class="Str"("Value"=w817) -> ()  [unwired: 2 in, 2 out]
            n416 = property on="WAGER TEAM 3" class="Str"("Value"=w817) -> ()  [unwired: 2 in, 2 out]
            n417 = Enqueue Element(queue=w832, element="WT1::0", error in (no error)=w831) -> (queue out=w827:refnum<queue>, error out=w826:errorcluster)  [unwired: 1 in, 1 out]
            n418 = property on="Is Daily Double or Final Jeopardy" class="Bool (strict)"("Value"=TRUE ("Is Daily Double or Final Jeopardy")) -> ()  [unwired: 2 in, 2 out]
            n419 = Enqueue Element(queue=w827, element="WT2::0", error in (no error)=w826) -> (queue out=w824:refnum<queue>, error out=w825:errorcluster)  [unwired: 1 in, 1 out]
            n420 = call <vilib>:"Open Config Data (compatibility).vi"("create file if necessary (T)"=FALSE ("create file if necessary? (T)"), "configuration file path"=w849) -> ("error out"=w845:errorcluster, "refnum"=w847:T3)  [unwired: 7 in, 1 out]
            n421 = call-poly <vilib>:"Read Key.vi"("section"=w838, "error in (no error)"=w845, "default value"="ERROR" ("key"), "key"="Question", "refnum"=w847) -> ("error out"=w841:errorcluster, "value"=w815:string, "refnum out"=w842:T3)  [unwired: 3 in, 1 out]
            n422 = Enqueue Element(queue=w824, element="WT3::0", error in (no error)=w825) -> (queue out=w822:refnum<queue>, error out=w821:errorcluster)  [unwired: 1 in, 1 out]
            n423 = property on="Question" class="Str"("Value"=w815) -> ()  [unwired: 2 in, 2 out]
            n424 = call-poly <vilib>:"Read Key.vi"("section"=w838, "error in (no error)"=w841, "default value"="ERROR" ("key"), "key"="Answer", "refnum"=w842) -> ("error out"=w840:errorcluster, "value"=w816:string, "refnum out"=w839:T3)  [unwired: 3 in, 1 out]
            n425 = property on="Answer" class="Str"("Value"=w816) -> ()  [unwired: 2 in, 2 out]
            n426 = call <vilib>:"Close Config Data.vi"("error in (no error)"=w840, "refnum"=w839) -> ("error out"=w843:errorcluster)  [unwired: 8 in, 1 out]
            n427 = property on="Special Answer" class="Str"("Value"=w816) -> ()  [unwired: 2 in, 2 out]
            n428 = property on="Special Question" class="Str"("Value"=w815) -> ()  [unwired: 2 in, 2 out]
            n429 = call <vilib>:"General Error Handler.vi"("error in (no error)"=w843) -> ()  [unwired: 10 in, 5 out]
            n430 = Enqueue Element(queue=w822, element="TAB::DIALOG", error in (no error)=w821) -> (queue out=w820:refnum<queue>, error out=w819:errorcluster)  [unwired: 1 in, 1 out]
          }
        }
      }
      event "Play/Display Question": Value Change {
        n431 = event-data() -> ("NewVal"=w868:bool)  [unwired: 1 in, 5 out]
        n432 = case shown="True" w868 {
          tunnel: w867 -> [w870 w880]
          tunnel: w866 -> [w869 w879]
          tunnel: [w870 w878] -> w865
          tunnel: [w869 w871] -> w864
          frame False {
          }
          frame True {
            n433 = property on="Question Setting" class="Ring (strict)"() -> ("Value"=w881:u16)  [unwired: 2 in, 2 out]
            n434 = property on="Category" class="DigNum (strict)"() -> ("Value"=w877:u8)  [unwired: 2 in, 2 out]
            n435 = property on="Question" class="DigNum (strict)"() -> ("Value"=w876:u8)  [unwired: 2 in, 2 out]
            n436 = property on="Play/Display Question" class="Bool (strict)"("Disabled"=u8 1) -> ()  [unwired: 2 in, 2 out]
            n437 = case shown="5" w876 {
              tunnel: [_ "QUESTION1" "QUESTION2" "QUESTION3" "QUESTION4" "QUESTION5" "QUESTION6"] -> w875
              frame 0, Default {
              }
              frame 1 {
              }
              frame 2 {
              }
              frame 3 {
              }
              frame 4 {
              }
              frame 5 {
              }
              frame 6 {
              }
            }
            n438 = case shown="7" w877 {
              tunnel: [_ w888 w889 w890 w891 w892 w893 w894] -> w874
              frame 0, Default {
              }
              frame 1 {
                n439 = property on="Category 1" class="Path"() -> ("Value"=w888:path)  [unwired: 2 in, 2 out]
              }
              frame 2 {
                n440 = property on="Category 2" class="Path"() -> ("Value"=w889:path)  [unwired: 2 in, 2 out]
              }
              frame 3 {
                n441 = property on="Category 3" class="Path"() -> ("Value"=w890:path)  [unwired: 2 in, 2 out]
              }
              frame 4 {
                n442 = property on="Category 4" class="Path"() -> ("Value"=w891:path)  [unwired: 2 in, 2 out]
              }
              frame 5 {
                n443 = property on="Category 5" class="Path"() -> ("Value"=w892:path)  [unwired: 2 in, 2 out]
              }
              frame 6 {
                n444 = property on="Category 6" class="Path"() -> ("Value"=w893:path)  [unwired: 2 in, 2 out]
              }
              frame 7 {
                n445 = property on="Final Jeopardy" class="Path"() -> ("Value"=w894:path)  [unwired: 2 in, 2 out]
              }
            }
            n446 = case shown="0, Default" w881 {
              tunnel: w880 -> [w907 w1092]
              tunnel: w879 -> [w906 w1091]
              tunnel: [w964 w1084] -> w878
              tunnel: [w963 w1083] -> w871
              tunnel: w875 -> [w946 _]
              tunnel: w874 -> [w938 w1070]
              frame 0, Default {
                w899 = 0 ("Button Pressed")
                n447 = Get Date/Time In Seconds() -> (seconds since 1Jan1904=w955:timestamp)
                n448 = Path to Array of Strings(0:w938) -> (2:w937:string[])  [unwired: 1 out]
                n449 = call <vilib>:"Open Config Data (compatibility).vi"("create file if necessary (T)"=FALSE ("create file if necessary? (T)"), "configuration file path"=w938) -> ("error out"=w960:errorcluster, "refnum"=w961:T3)  [unwired: 7 in, 1 out]
                n450 = Get Date/Time String(seconds (now)=w955) -> (date string=w954:string, time string=w953:string)  [unwired: 2 in]
                n451 = Array Size(array=w937) -> (size(s)=w931:i32)
                n452 = property on="Timeout" class="Bool (strict)"("Value"=TRUE ("Timeout")) -> (error out=w908:errorcluster)  [unwired: 2 in, 1 out]
                n453 = property on="Team Pressed" class="DigNum (strict)"("Value"=w899) -> (error out=w900:errorcluster)  [unwired: 2 in, 1 out]
                n454 = property on="Button Pressed" class="DigNum (strict)"("Value"=w899) -> (error out=w912:errorcluster)  [unwired: 2 in, 1 out]
                n455 = Concatenate Strings(w954, " " ("string"), w953) -> (w951:string)
                n456 = call-poly <vilib>:"Write Key.vi"("section"="HEADER", "error in (no error)"=w960, "value"=w951, "key"="Used", "refnum"=w961) -> ("error out"=w957:errorcluster, "refnum out"=w956:T3)  [unwired: 4 in, 1 out]
                n457 = flat-sequence {
                  tunnel: w944 -> [w1038]
                  tunnel: w943 -> [w1037]
                  tunnel: [w1036] -> w930
                  tunnel: [w1035] -> w929
                  tunnel: w922 -> [w1034]
                  tunnel: [w1034] -> w921
                  tunnel: [w1033] -> w920
                  tunnel: w912 -> [w1032]
                  tunnel: [w1032] -> w911
                  tunnel: w908 -> [_]
                  tunnel: w900 -> [_]
                  frame #0 {
                    n458 = Tick Count (ms)() -> (millisecond timer value=w1033:u32)
                    n459 = call <vilib>:"SO Start.vi"("error in (no error)"=w1038, "task ID in"=w1037) -> ("error out"=w1035:errorcluster, "task ID out"=w1036:u32)  [unwired: 8 in]
                  }
                }
                n460 = Decrement(x=w931) -> (x-1=w932:i32)
                n461 = Array Subset(array=w937, length=w932) -> (w936:string[])  [unwired: 1 in]
                n462 = case shown="No Error" w929 {
                  selector: w929 -> [_ w1062]
                  tunnel: w930 -> [w1046 w1063]
                  tunnel: [w1045 w1063] -> w927
                  tunnel: [_ w1062] -> w928
                  tunnel: w921 -> [w1044 _]
                  tunnel: w920 -> [w1043 _]
                  tunnel: [w1042 TRUE] -> w903
                  tunnel: [w1041 0] -> _
                  tunnel: w911 -> [w1040 w1060]
                  tunnel: [w1039 w1060] -> w910
                  frame No Error {
                    n463 = while {
                      tunnel: w1046 -> [w1058]
                      tunnel: [w1058] -> w1045
                      tunnel: w1044 -> [w1054]
                      tunnel: w1043 -> [w1056]
                      tunnel: [w1050] -> w1042
                      tunnel: [w1052] -> w1041
                      tunnel: w1040 -> [w1051]
                      tunnel: [w1051] -> w1039
                      stop <- w1049 stop-if-true
                      n464 = property on="Button Pressed" class="DigNum (strict)"() -> ("Value"=w1052:i32)  [unwired: 2 in, 2 out]
                      n465 = Tick Count (ms)() -> (millisecond timer value=w1057:u32)
                      n466 = Not Equal?(x=w1052, y=0) -> (x != y?=w1050:bool)
                      n467 = Subtract(x=w1057, y=w1056) -> (x-y=w1055:u32)
                      n468 = Greater Or Equal?(x=w1055, y=w1054) -> (x >= y?=w1048:bool)
                      n469 = property on="stop" class="Bool (strict)"() -> ("Value"=w1047:bool)  [unwired: 2 in, 2 out]
                      n470 = Compound Arithmetic op=OR(w1047, w1048, w1050) -> (w1049:bool)
                    }
                  }
                  frame Error {
                  }
                }
                n471 = call-poly <vilib>:"Read Key.vi"("section"=w946, "error in (no error)"=w957, "default value"="ERROR" ("key"), "key"="Recording", "refnum"=w956) -> ("error out"=w947:errorcluster, "value"=w935:string, "refnum out"=w948:T3)  [unwired: 3 in, 1 out]
                n472 = property on="Final Jeopardy Time" class="DigNum (strict)"() -> ("Value"=w897:u8)  [unwired: 2 in, 2 out]
                n473 = Insert Into Array(array=w936, new element=w935) -> (w934:string[])  [unwired: 1 in]
                n474 = call <vilib>:"Close Config Data.vi"("error in (no error)"=w947, "refnum"=w948) -> ("error out"=w939:errorcluster)  [unwired: 8 in, 1 out]
                n475 = property on="Is Daily Double or Final Jeopardy" class="Bool (strict)"() -> ("Value"=w898:bool)  [unwired: 2 in, 2 out]
                n476 = Array of Strings to Path(0:w934) -> (2:w933:path)  [unwired: 1 in]
                n477 = call <vilib>:"Snd Read Wave File.vi"("wave file path"=w933) -> ("error out"=w940:errorcluster, "sound format"=w917:T4, "mono 16-bit"=w926:i16[])  [unwired: 4 in, 4 out]
                n478 = Unbundle By Name(w917) -> ("rate"=w916:enum16{"11025", "22050", "44100", "8000"})
                n479 = Array Size(array=w926) -> (size(s)=w919:i32)
                n480 = case shown="\"44100\"" w916 {
                  tunnel: [11025.0 ("y") 22050.0 ("y") 44100.0 ("y") 8000.0 ("y")] -> w915
                  frame "11025", Default {
                  }
                  frame "22050" {
                  }
                  frame "44100" {
                  }
                  frame "8000" {
                  }
                }
                n481 = To Double Precision Float(number=w919) -> (double precision float=w918:dbl)
                n482 = call <vilib>:"SO Config.vi"("error in (no error)"=w940, "sound format"=w917) -> ("error out"=w941:errorcluster, "task ID out"=w942:u32)  [unwired: 8 in]
                n483 = call <vilib>:"SO Write.vi"("mono 16-bit"=w926, "error in (no error)"=w941, "task ID in"=w942) -> ("error out"=w944:errorcluster, "task ID out"=w943:u32)  [unwired: 7 in]
                n484 = Divide(x=w918, y=w915) -> (x/y=w925:dbl)
                n485 = Multiply(x=w925, y=1000.0) -> (x*y=w923:dbl)
                n486 = To Unsigned Long Integer(number=w923) -> (unsigned 32bit integer=w922:u32)
                n487 = property on="Question Time" class="DigNum (strict)"() -> ("Value"=w901:u8)  [unwired: 2 in, 2 out]
                n488 = case shown="False" w898 {
                  tunnel: [w982 w1008] -> w895
                  tunnel: w910 -> [w981 w1008]
                  tunnel: w907 -> [w980 w1007]
                  tunnel: w906 -> [w979 w1006]
                  tunnel: [w978 w1004] -> w905
                  tunnel: [w977 w1005] -> w904
                  tunnel: w903 -> [w976 w1009]
                  tunnel: [w975 w1009] -> w902
                  tunnel: w901 -> [w974 _]
                  tunnel: w897 -> [_ w999]
                  frame False {
                    n489 = case shown="False" w976 {
                      selector: w976 -> [w987 w997]
                      tunnel: [w994 w998] -> w982
                      tunnel: w981 -> [w992 w998]
                      tunnel: w980 -> [w991 w996]
                      tunnel: w979 -> [w990 w995]
                      tunnel: [w988 w996] -> w978
                      tunnel: [w989 w995] -> w977
                      tunnel: [w987 w997] -> w975
                      tunnel: w974 -> [w983 _]
                      frame False {
                        n490 = Number To Decimal String(number=w983) -> (decimal integer string=w984:string)  [unwired: 1 in]
                        n491 = Concatenate Strings("TIMER" ("string"), w984) -> (w985:string)
                        n492 = Enqueue Element(queue=w991, element=w985, error in (no error)=w990) -> (queue out=w988:refnum<queue>, error out=w989:errorcluster)  [unwired: 1 in, 1 out]
                        n493 = call "SendMsg.vi"("Data"="$S00", "error in (no error)"=w992) -> ("error out"=w994:errorcluster)  [unwired: 13 in]
                      }
                      frame True {
                      }
                    }
                  }
                  frame True {
                    n494 = Number To Decimal String(number=w999) -> (decimal integer string=w1002:string)  [unwired: 1 in]
                    n495 = property on="Is Daily Double or Final Jeopardy" class="Bool (strict)"("Value"=FALSE ("Is Final Jeopardy")) -> ()  [unwired: 2 in, 2 out]
                    n496 = Concatenate Strings("TIMER" ("string"), w1002) -> (w1001:string)
                    n497 = Enqueue Element(queue=w1007, element=w1001, error in (no error)=w1006) -> (queue out=w1004:refnum<queue>, error out=w1005:errorcluster)  [unwired: 1 in, 1 out]
                  }
                }
                n498 = call <vilib>:"SO Stop.vi"("error in (no error)"=w928, "task ID in"=w927) -> ("error out"=w914:errorcluster, "task ID out"=w945:u32)  [unwired: 8 in]
                n499 = call <vilib>:"SI Clear.vi"("error in (no error)"=w914, "task ID in"=w945) -> ("error out"=w913:errorcluster)  [unwired: 9 in]
                n500 = while {
                  tunnel: w895 -> [_]
                  stop <- w1012 stop-if-true
                  n501 = property on="Button Pressed" class="DigNum (strict)"() -> ("Value"=w1014:i32)  [unwired: 2 in, 2 out]
                  n502 = property on="Timeout" class="Bool (strict)"() -> ("Value"=w1011:bool)  [unwired: 2 in, 2 out]
                  n503 = Not Equal?(x=w1014, y=0 ("length (rest)")) -> (x != y?=w1013:bool)
                  n504 = property on="stop" class="Bool (strict)"() -> ("Value"=w1010:bool)  [unwired: 2 in, 2 out]
                  n505 = Compound Arithmetic op=OR(w1010, w1011, w1013) -> (w1012:bool)
                }
                n506 = case shown="False" w902 {
                  tunnel: w904 -> [w1025 w1026]
                  tunnel: [w1017 w1027] -> w964
                  tunnel: [w1016 w1026] -> w963
                  tunnel: w905 -> [w1024 w1027]
                  tunnel: w913 -> [_ _]
                  frame False {
                    n507 = property on="Question" class="Str"() -> ("Value"=w1023:string)  [unwired: 2 in, 2 out]
                    n508 = Enqueue Element(queue=w1024, element="A::::", error in (no error)=w1025) -> (queue out=w1020:refnum<queue>, error out=w1019:errorcluster)  [unwired: 1 in, 1 out]
                    n509 = Concatenate Strings("Q::::" ("string"), w1023) -> (w1022:string)
                    n510 = Enqueue Element(queue=w1020, element=w1022, error in (no error)=w1019) -> (queue out=w1017:refnum<queue>, error out=w1016:errorcluster)  [unwired: 1 in, 1 out]
                  }
                  frame True {
                  }
                }
                n511 = Merge Errors(w939, w913, w895) -> (w896:errorcluster)
                n512 = case shown="No Error" w895 {
                  tunnel: w896 -> [w965 w973]
                  frame No Error {
                    n513 = call <vilib>:"General Error Handler.vi"("error in (no error)"=w965) -> ()  [unwired: 10 in, 5 out]
                  }
                  frame Error {
                    n514 = Unbundle By Name(w973) -> ("status"=w967:bool, "code"=w966:i32, "source"=w970:string)
                    n515 = Concatenate Strings(w970, "\r", "DID YOU PICK A NEW QUESTION?") -> (w971:string)
                    n516 = Bundle By Name(cluster=w973, "status"=w967, "code"=w966, "source"=w971) -> (w972:errorcluster)
                    n517 = call <vilib>:"General Error Handler.vi"("error in (no error)"=w972) -> ()  [unwired: 10 in, 5 out]
                  }
                }
              }
              frame 1 {
                n518 = Get Date/Time In Seconds() -> (seconds since 1Jan1904=w1075:timestamp)
                n519 = property on="Is Daily Double or Final Jeopardy" class="Bool (strict)"() -> ("Value"=w1067:bool)  [unwired: 2 in, 2 out]
                n520 = call <vilib>:"Open Config Data (compatibility).vi"("create file if necessary (T)"=FALSE ("create file if necessary? (T)"), "configuration file path"=w1070) -> ("error out"=w1078:errorcluster, "refnum"=w1079:T3)  [unwired: 7 in, 1 out]
                n521 = Get Date/Time String(seconds (now)=w1075) -> (date string=w1074:string, time string=w1073:string)  [unwired: 2 in]
                n522 = Concatenate Strings(w1074, " " ("string"), w1073) -> (w1071:string)
                n523 = case shown="False" w1067 {
                  tunnel: [w1105 _] -> w1064
                  frame False {
                    n524 = call "SendMsg.vi"("Data"="$S00") -> ("error out"=w1105:errorcluster)  [unwired: 14 in]
                  }
                  frame True {
                    n525 = property on="Is Daily Double or Final Jeopardy" class="Bool (strict)"("Value"=FALSE ("Is Final Jeopardy")) -> ()  [unwired: 2 in, 2 out]
                  }
                }
                n526 = call-poly <vilib>:"Write Key.vi"("section"="HEADER", "error in (no error)"=w1078, "value"=w1071, "key"="Used", "refnum"=w1079) -> ("error out"=w1068:errorcluster, "refnum out"=w1069:T3)  [unwired: 4 in, 1 out]
                n527 = call <vilib>:"Close Config Data.vi"("error in (no error)"=w1068, "refnum"=w1069) -> ("error out"=w1065:errorcluster)  [unwired: 8 in, 1 out]
                n528 = Enqueue Element(queue=w1092, element="A::::", error in (no error)=w1091) -> (queue out=w1089:refnum<queue>, error out=w1090:errorcluster)  [unwired: 1 in, 1 out]
                n529 = property on="Question" class="Str"() -> ("Value"=w1096:string)  [unwired: 2 in, 2 out]
                n530 = while {
                  tunnel: w1064 -> [_]
                  stop <- w1109 stop-if-true
                  n531 = property on="Button Pressed" class="DigNum (strict)"() -> ("Value"=w1111:i32)  [unwired: 2 in, 2 out]
                  n532 = property on="Timeout" class="Bool (strict)"() -> ("Value"=w1108:bool)  [unwired: 2 in, 2 out]
                  n533 = Not Equal?(x=w1111, y=0 ("length (rest)")) -> (x != y?=w1110:bool)
                  n534 = property on="stop" class="Bool (strict)"() -> ("Value"=w1107:bool)  [unwired: 2 in, 2 out]
                  n535 = Compound Arithmetic op=OR(w1107, w1108, w1110) -> (w1109:bool)
                }
                n536 = Concatenate Strings("Q::::" ("string"), w1096) -> (w1095:string)
                n537 = Enqueue Element(queue=w1089, element=w1095, error in (no error)=w1090) -> (queue out=w1082:refnum<queue>, error out=w1081:errorcluster)  [unwired: 1 in, 1 out]
                n538 = Merge Errors(w1065, w1064) -> (w1066:errorcluster)
                n539 = case shown="Error" w1064 {
                  tunnel: w1066 -> [w1097 w1098]
                  frame No Error {
                    n540 = call <vilib>:"General Error Handler.vi"("error in (no error)"=w1097) -> ()  [unwired: 10 in, 5 out]
                  }
                  frame Error {
                    n541 = Unbundle By Name(w1098) -> ("source"=w1101:string)
                    n542 = Concatenate Strings(w1101, "\r", "DID YOU PICK A NEW QUESTION?") -> (w1102:string)
                    n543 = Bundle By Name(cluster=w1098, "source"=w1102) -> (w1103:errorcluster)
                    n544 = call <vilib>:"General Error Handler.vi"("error in (no error)"=w1103) -> ()  [unwired: 10 in, 5 out]
                  }
                }
                n545 = property on="Question Time" class="DigNum (strict)"() -> ("Value"=w1085:u8)  [unwired: 2 in, 2 out]
                n546 = Number To Decimal String(number=w1085) -> (decimal integer string=w1086:string)  [unwired: 1 in]
                n547 = Concatenate Strings("TIMER" ("string"), w1086) -> (w1087:string)
                n548 = Enqueue Element(queue=w1082, element=w1087, error in (no error)=w1081) -> (queue out=w1084:refnum<queue>, error out=w1083:errorcluster)  [unwired: 1 in, 1 out]
              }
            }
            n549 = property on="Play/Display Question" class="Bool (strict)"(error in=w871, "Disabled"=u8 0) -> ()  [unwired: 1 in, 2 out]
          }
        }
      }
      event "Play/Display": Value Change {
        n550 = event-data() -> ("NewVal"=w1113:bool)  [unwired: 1 in, 5 out]
        n551 = case shown="True" w1113 {
          frame False {
          }
          frame True {
            n552 = property on="Teams" class="Ring (strict)"() -> ("Value"=w1115:u16)  [unwired: 2 in, 2 out]
            n553 = property on="Play/Display Question" class="Bool (strict)"("Value (Signaling)"=TRUE) -> (error out=w1116:errorcluster)  [unwired: 2 in, 1 out]
            n554 = case shown="0, Default" w1115 {
              frame 1 {
                w1119 = TRUE ("Visible")
                n555 = property on="Team 1 W/R?" class="Bool (strict)"("Visible"=w1119) -> ()  [unwired: 2 in, 2 out]
                n556 = property on="Team 2 W/R?" class="Bool (strict)"("Visible"=w1119) -> ()  [unwired: 2 in, 2 out]
                n557 = property on="Team 3 W/R?" class="Bool (strict)"("Visible"=w1119) -> ()  [unwired: 2 in, 2 out]
              }
              frame 0, Default {
                w1120 = TRUE ("Visible")
                n558 = property on="Team 1 W/R?" class="Bool (strict)"("Visible"=w1120) -> ()  [unwired: 2 in, 2 out]
                n559 = property on="Team 2 W/R?" class="Bool (strict)"("Visible"=w1120) -> ()  [unwired: 2 in, 2 out]
              }
            }
            n560 = property on="Play/Display Question" class="Bool (strict)"(error in=w1116, "Value"=FALSE ("Play/Display Question")) -> ()  [unwired: 1 in, 2 out]
            n561 = property on="Dialog Done" class="Bool (strict)"("Visible"=TRUE) -> ()  [unwired: 2 in, 2 out]
          }
        }
      }
      event "Final Jeopardy": Value Change {
        n562 = event-data() -> ("NewVal"=w1126:bool)  [unwired: 1 in, 5 out]
        n563 = property on="Final Jeopardy" class="Bool (strict)"("Value"=FALSE ("Final Jeopardy")) -> ()  [unwired: 2 in, 2 out]
        n564 = case shown="True" w1126 {
          tunnel: w1125 -> [w1128 w1154]
          tunnel: w1124 -> [w1127 w1153]
          tunnel: [w1128 w1152] -> w1123
          tunnel: [w1127 w1151] -> w1122
          frame False {
          }
          frame True {
            w1133 = "QUESTION5"
            w1137 = "0" ("WAGER TEAM 1")
            n565 = property on="Final Jeopardy" class="Path"() -> ("Value"=w1132:path)  [unwired: 2 in, 2 out]
            n566 = property on="Is Daily Double or Final Jeopardy" class="Bool (strict)"("Value"=TRUE ("Is Final Jeopardy")) -> ()  [unwired: 2 in, 2 out]
            n567 = property on="Tab Control" class="TabCtl (strict)"("Value"=T2."Wager Dialog" ("Tab Control")) -> ()  [unwired: 2 in, 2 out]
            n568 = property on="Dialog Done" class="Bool (strict)"("Visible"=FALSE) -> ()  [unwired: 2 in, 2 out]
            n569 = Enqueue Element(queue=w1154, element="DIAL:FINAL JEOPARDY", error in (no error)=w1153) -> (queue out=w1166:refnum<queue>, error out=w1165:errorcluster)  [unwired: 1 in, 1 out]
            n570 = property on="Category" class="DigNum (strict)"("Value"=u8 7 ("Category")) -> ()  [unwired: 2 in, 2 out]
            n571 = property on="Question" class="DigNum (strict)"("Value"=u8 5 ("Question")) -> ()  [unwired: 2 in, 2 out]
            n572 = property on="WAGER TEAM 1" class="Str"("Value"=w1137) -> ()  [unwired: 2 in, 2 out]
            n573 = property on="WAGER TEAM 2" class="Str"("Value"=w1137) -> ()  [unwired: 2 in, 2 out]
            n574 = property on="WAGER TEAM 3" class="Str"("Value"=w1137) -> ()  [unwired: 2 in, 2 out]
            n575 = Enqueue Element(queue=w1166, element="WT1::0", error in (no error)=w1165) -> (queue out=w1161:refnum<queue>, error out=w1160:errorcluster)  [unwired: 1 in, 1 out]
            n576 = call <vilib>:"Open Config Data (compatibility).vi"("create file if necessary (T)"=FALSE ("create file if necessary? (T)"), "configuration file path"=w1132) -> ("error out"=w1147:errorcluster, "refnum"=w1149:T3)  [unwired: 7 in, 1 out]
            n577 = Enqueue Element(queue=w1161, element="WT2::0", error in (no error)=w1160) -> (queue out=w1158:refnum<queue>, error out=w1159:errorcluster)  [unwired: 1 in, 1 out]
            n578 = call-poly <vilib>:"Read Key.vi"("section"=w1133, "error in (no error)"=w1147, "default value"="ERROR" ("key"), "key"="Question", "refnum"=w1149) -> ("error out"=w1143:errorcluster, "value"=w1135:string, "refnum out"=w1144:T3)  [unwired: 3 in, 1 out]
            n579 = property on="Question" class="Str"("Value"=w1135) -> ()  [unwired: 2 in, 2 out]
            n580 = call-poly <vilib>:"Read Key.vi"("section"=w1133, "error in (no error)"=w1143, "default value"="ERROR" ("key"), "key"="Answer", "refnum"=w1144) -> ("error out"=w1142:errorcluster, "value"=w1136:string, "refnum out"=w1141:T3)  [unwired: 3 in, 1 out]
            n581 = Enqueue Element(queue=w1158, element="WT3::0", error in (no error)=w1159) -> (queue out=w1156:refnum<queue>, error out=w1155:errorcluster)  [unwired: 1 in, 1 out]
            n582 = property on="Answer" class="Str"("Value"=w1136) -> ()  [unwired: 2 in, 2 out]
            n583 = call <vilib>:"Close Config Data.vi"("error in (no error)"=w1142, "refnum"=w1141) -> ("error out"=w1145:errorcluster)  [unwired: 8 in, 1 out]
            n584 = property on="Special Answer" class="Str"("Value"=w1136) -> ()  [unwired: 2 in, 2 out]
            n585 = property on="Special Question" class="Str"("Value"=w1135) -> ()  [unwired: 2 in, 2 out]
            n586 = call <vilib>:"General Error Handler.vi"("error in (no error)"=w1145) -> ()  [unwired: 10 in, 5 out]
            n587 = Enqueue Element(queue=w1156, element="TAB::DIALOG", error in (no error)=w1155) -> (queue out=w1152:refnum<queue>, error out=w1151:errorcluster)  [unwired: 1 in, 1 out]
          }
        }
      }
    }
  }
  n588 = while {
    tunnel: w66 -> [w1177]
    tunnel: w65 -> [w1178]
    tunnel: [w1171] -> w64
    tunnel: [w1170] -> w63
    tunnel: bool[][] [[FALSE, FALSE, FALSE, FALSE, FALSE, FALSE], [FALSE, FALSE, FALSE, FALSE, FALSE, FALSE], [FALSE, FALSE, FALSE, FALSE, FALSE, FALSE], [FALSE, FALSE, FALSE, FALSE, FALSE, FALSE], [FALSE, FALSE, FALSE, FALSE, FALSE, FALSE]] ("GameGUI") -> [w1168]
    stop <- w1169 stop-if-true
    n589 = Dequeue Element(queue=w1178, timeout in ms (-1)=100, error in (no error)=w1177) -> (queue out=w1174:refnum<queue>, element=w1172:string, timed out?=w1175:bool, error out=w1173:errorcluster)
    n590 = case shown="False" w1175 {
      tunnel: w1174 -> [w1186 w1236]
      tunnel: w1173 -> [w1187 w1235]
      tunnel: w1172 -> [w1180 _]
      tunnel: [w1185 w1236] -> w1171
      tunnel: [w1184 w1235] -> w1170
      tunnel: w1168 -> [w1179 _]
      frame False {
        n591 = String Subset(string=w1180, offset (0)=0, length (rest)=4 ("length (rest)")) -> (substring=w1183:string)
        n592 = case shown="\"BTNP\"" w1183 {
          tunnel: w1187 -> [w1226 w1233]
          tunnel: w1186 -> [w1227 w1234]
          tunnel: [w1227 w1234] -> w1185
          tunnel: [w1226 w1233] -> w1184
          tunnel: w1180 -> [w1225 _]
          tunnel: w1179 -> [w1224 _]
          frame "BTNP" {
            n593 = property on="Question" class="DigNum (strict)"() -> ("Value"=w1209:u8)  [unwired: 2 in, 2 out]
            n594 = property on="Category" class="DigNum (strict)"() -> ("Value"=w1208:u8)  [unwired: 2 in, 2 out]
            n595 = property on="Daily Double Questions" class="Arr (strict)"() -> ("Value"=w1218:i32[])  [unwired: 2 in, 2 out]
            n596 = property on="Daily Double Categories" class="Arr (strict)"() -> ("Value"=w1210:i32[])  [unwired: 2 in, 2 out]
            n597 = Index Array(array=w1218, index #1=0 ("index"), index #2=1 ("index")) -> (element #1=w1220:i32, element #2=w1221:i32)
            n598 = Index Array(array=w1210, index #1=0 ("index"), index #2=1 ("index")) -> (element #1=w1213:i32, element #2=w1214:i32)
            n599 = Equal?(x=w1220, y=w1209) -> (x = y?=w1222:bool)
            n600 = Equal?(x=w1221, y=w1209) -> (x = y?=w1223:bool)
            n601 = Equal?(x=w1213, y=w1208) -> (x = y?=w1215:bool)
            n602 = Equal?(x=w1214, y=w1208) -> (x = y?=w1216:bool)
            n603 = Or(x=w1222, y=w1223) -> (x .or. y?=w1207:bool)
            n604 = Or(x=w1215, y=w1216) -> (x .or. y?=w1206:bool)
            n605 = And(x=w1207, y=w1206) -> (x .and. y?=w1190:bool)
            n606 = property on="Game Started" class="Bool (strict)"() -> ("Value"=w1191:bool)  [unwired: 2 in, 2 out]
            n607 = Not(x=w1190) -> (.not. x?=w1189:bool)
            n608 = String Subset(string=w1225, offset (0)=5, length (rest)=1 ("length (rest)")) -> (substring=w1202:string)
            n609 = String Subset(string=w1225, offset (0)=4, length (rest)=1 ("length (rest)")) -> (substring=w1201:string)
            n610 = And(x=w1189, y=w1191) -> (x .and. y?=w1188:bool)
            n611 = Decimal String To Number(string=w1202) -> (number=w1195:i32)  [unwired: 2 in, 1 out]
            n612 = Decimal String To Number(string=w1201) -> (number=w1196:i32)  [unwired: 2 in, 1 out]
            n613 = Decrement(x=w1195) -> (x-1=w1197:i32)
            n614 = Decrement(x=w1196) -> (x-1=w1198:i32)
            n615 = property on="Question" class="DigNum (strict)"("Value"=w1195) -> (error out=w1193:errorcluster)  [unwired: 2 in, 1 out]
            n616 = property on="Category" class="DigNum (strict)"("Value"=w1196) -> (error out=w1192:errorcluster)  [unwired: 2 in, 1 out]
            n617 = Replace Array Subset(array=w1224, new element=TRUE ("new element/subarray"), index (row)=w1197, index (col)=w1198) -> (w1194:bool[][])
            n618 = flat-sequence {
              tunnel: w1194 -> [w1229]
              tunnel: w1193 -> [_]
              tunnel: w1192 -> [_]
              tunnel: w1188 -> [w1228]
              frame #0 {
                n619 = property on="GameGUI" class="Arr (strict)"("Value (Signaling)"=w1229) -> ()  [unwired: 2 in, 2 out]
                n620 = case shown="True" w1228 {
                  frame False {
                  }
                  frame True {
                    n621 = property on="WRONG" class="Bool (strict)"("Disabled"=u8 1) -> ()  [unwired: 2 in, 2 out]
                    n622 = property on="RIGHT" class="Bool (strict)"("Disabled"=u8 1) -> ()  [unwired: 2 in, 2 out]
                    n623 = call "SendMsg.vi"("Data"="$E00") -> ()  [unwired: 14 in, 1 out]
                  }
                }
              }
            }
          }
          frame Default {
          }
        }
        "Received Message" <- w1180
      }
      frame True {
      }
    }
    n624 = property on="stop" class="Bool (strict)"() -> ("Value"=w1169:bool)  [unwired: 2 in, 2 out]
  }
  n625 = while {
    tunnel: w30 -> [w1243]
    tunnel: w29 -> [w1244]
    shift-right: [w1246] -> w21
    shift-left: errorcluster {"status"=TRUE, "code"=1000, "source"="Cannot Open Com Port"} ("error out") -> [w1248]
    shift-right: [w1247] -> w26
    shift-left: refnum<visa-resource-name> "COM1" ("COM Port") -> [w1245]
    tunnel: [w1242] -> w25
    tunnel: [w1241] -> w24
    tunnel: w15 -> [w1240]
    tunnel: w14 -> [w1239]
    tunnel: [w1238] -> w13
    tunnel: [w1237] -> w12
    stop <- w1249 stop-if-true
    n626 = case shown="No Error" w1248 {
      selector: w1248 -> [w1282 _]
      tunnel: [w1267 w1484] -> w1247
      tunnel: [w1266 w1483] -> w1246
      tunnel: w1245 -> [w1283 _]
      tunnel: w1244 -> [w1281 w1482]
      tunnel: w1243 -> [w1280 w1481]
      tunnel: [w1262 w1481] -> w1241
      tunnel: [w1263 w1482] -> w1242
      tunnel: w1240 -> [w1255 w1480]
      tunnel: w1239 -> [w1254 w1479]
      tunnel: [w1253 w1480] -> w1238
      tunnel: [w1252 w1479] -> w1237
      frame No Error {
        n627 = property on="Com Msgs" class="Str"() -> ("Value"=w1259:string)  [unwired: 2 in, 2 out]
        n628 = Dequeue Element(queue=w1281, timeout in ms (-1)=5, error in (no error)=w1280) -> (queue out=w1279:refnum<queue>, element=w1275:string, timed out?=w1278:bool, error out=w1276:errorcluster)
        n629 = case shown="False" w1278 {
          tunnel: w1283 -> [w1432 w1476]
          tunnel: w1282 -> [w1431 w1475]
          tunnel: w1279 -> [w1430 w1478]
          tunnel: w1276 -> [w1429 w1477]
          tunnel: w1275 -> [w1414 _]
          tunnel: [w1430 w1478] -> w1265
          tunnel: [w1429 w1477] -> w1264
          tunnel: [w1425 w1476] -> w1273
          tunnel: [w1426 w1475] -> w1274
          tunnel: "Received incorrect validation for " ("source") -> [w1417 _]
          tunnel: "Received invalid for " ("source") -> [w1416 _]
          tunnel: w1259 -> [w1415 w1474]
          tunnel: [w1412 w1474] -> w1258
          tunnel: " DID YOU PICK A NEW QUESTION?" ("source") -> [w1410 _]
          tunnel: " YOU PROBABLY FORGOT TO CLICK \"START GAME\"?\n TRY TO CONTINUE GAME PLAY." ("source") -> [w1409 _]
          frame False {
            n630 = VISA Write(VISA resource name=w1432, write buffer=w1414, error in (no error)=w1431) -> (VISA resource name out=w1428:refnum<visa-resource-name>, error out=w1427:errorcluster)  [unwired: 1 out]
            n631 = String Subset(string=w1414, offset (0)=1, length (rest)=1 ("length (rest)")) -> (substring=w1418:string)
            n632 = VISA Read(VISA resource name=w1428, byte count=u32 5, error in (no error)=w1427) -> (VISA resource name out=w1425:refnum<visa-resource-name>, read buffer=w1413:string, error out=w1426:errorcluster)  [unwired: 1 out]
            n633 = String Subset(string=w1413, offset (0)=0, length (rest)=2 ("length (rest)")) -> (substring=w1421:string)
            n634 = Concatenate Strings(w1415, w1414, w1413, "\r") -> (w1412:string)
            n635 = case shown="\"$I\"" w1421 {
              tunnel: w1413 -> [_ _ w1469]
              tunnel: w1418 -> [_ _ w1465]
              tunnel: w1417 -> [_ _ w1462]
              tunnel: w1414 -> [w1435 w1455 w1461]
              tunnel: w1416 -> [w1437 _ _]
              tunnel: w1410 -> [w1434 _ _]
              tunnel: w1409 -> [w1433 _ _]
              frame "$I" {
                n636 = Wait (ms)(milliseconds to wait=u32 500) -> ()  [unwired: 1 out]
                n637 = property on="Communication" class="Bool (strict)"("Value"=FALSE ("Communication")) -> ()  [unwired: 2 in, 2 out]
                n638 = case shown="\"$E00\"" w1435 {
                  tunnel: w1435 -> [w1445 w1449 w1453]
                  tunnel: w1437 -> [w1444 w1448 w1452]
                  tunnel: [w1443 w1447 w1451] -> w1436
                  tunnel: w1434 -> [_ w1446 _]
                  tunnel: w1433 -> [_ _ w1450]
                  frame Default {
                    n639 = Concatenate Strings(w1444, w1445) -> (w1443:string)
                  }
                  frame "$S00" {
                    n640 = Concatenate Strings(w1448, w1449, w1446) -> (w1447:string)
                  }
                  frame "$E00" {
                    n641 = Concatenate Strings(w1452, w1453, w1450) -> (w1451:string)
                  }
                }
                n642 = Bundle("status"=TRUE, "code"=1000, w1436) -> (w1440:cluster{"status":bool, "code":i32, string})  [unwired: 1 in]
                n643 = call <vilib>:"General Error Handler.vi"("error in (no error)"=w1440) -> ()  [unwired: 10 in, 5 out]
              }
              frame Default {
                n644 = Concatenate Strings("Did not receive response for " ("source"), w1455) -> (w1454:string)
                n645 = Bundle("status"=TRUE, "code"=1000, w1454) -> (w1459:cluster{"status":bool, "code":i32, string})  [unwired: 1 in]
                n646 = call <vilib>:"General Error Handler.vi"("error in (no error)"=w1459) -> ()  [unwired: 10 in, 5 out]
              }
              frame "$V" {
                n647 = String Subset(string=w1469, offset (0)=3, length (rest)=1 ("length (rest)")) -> (substring=w1466:string)
                n648 = property on="Communication" class="Bool (strict)"("Value"=TRUE ("Communication")) -> ()  [unwired: 2 in, 2 out]
                n649 = Equal?(x=w1465, y=w1466) -> (x = y?=w1463:bool)
                n650 = Concatenate Strings(w1462, w1461) -> (w1460:string)
                n651 = case shown="False" w1463 {
                  tunnel: w1460 -> [w1470 _]
                  frame False {
                    n652 = Bundle("status"=TRUE, "code"=1000, w1470) -> (w1473:cluster{"status":bool, "code":i32, string})  [unwired: 1 in]
                    n653 = call <vilib>:"General Error Handler.vi"("error in (no error)"=w1473) -> ()  [unwired: 10 in, 5 out]
                  }
                  frame True {
                  }
                }
              }
            }
          }
          frame True {
          }
        }
        n654 = property on="Com Msgs" class="Str"("Value"=w1258) -> ()  [unwired: 2 in, 2 out]
        n655 = property class="Instr"(reference=w1273, error in=w1274) -> (reference out=w1272:refnum<visa-resource-name>, error out=w1271:errorcluster, "Serial Settings:Number of Bytes at Serial Port"=w1269:u32)
        n656 = property on="Com Msgs" class="Str"() -> ("Value"=w1257:string)  [unwired: 2 in, 2 out]
        n657 = Greater Or Equal?(x=w1269, y=u32 5) -> (x >= y?=w1270:bool)
        n658 = case shown="True" w1270 {
          tunnel: w1272 -> [w1290 w1310]
          tunnel: w1271 -> [w1289 w1309]
          tunnel: [w1290 w1301] -> w1267
          tunnel: [w1289 w1300] -> w1266
          tunnel: w1265 -> [w1288 w1308]
          tunnel: w1264 -> [w1287 w1307]
          tunnel: [w1288 w1308] -> w1263
          tunnel: [w1287 w1307] -> w1262
          tunnel: [_ w1297] -> _
          tunnel: w1257 -> [w1286 w1299]
          tunnel: [w1286 w1296] -> w1256
          tunnel: w1255 -> [w1285 w1294]
          tunnel: w1254 -> [w1284 w1293]
          tunnel: [w1285 w1292] -> w1253
          tunnel: [w1284 w1291] -> w1252
          frame False {
          }
          frame True {
            n659 = VISA Read(VISA resource name=w1310, byte count=u32 5, error in (no error)=w1309) -> (VISA resource name out=w1303:refnum<visa-resource-name>, read buffer=w1298:string, error out=w1302:errorcluster)  [unwired: 1 out]
            n660 = String Subset(string=w1298, offset (0)=0, length (rest)=2 ("length (rest)")) -> (substring=w1304:string)
            n661 = case shown="\"$N\"" w1304 {
              tunnel: w1303 -> [w1321 w1337 w1353 w1365 w1374 w1404]
              tunnel: w1302 -> [w1320 w1336 w1352 w1364 w1373 w1403]
              tunnel: [w1322 w1339 w1355 w1367 w1375 w1402] -> w1301
              tunnel: [w1323 w1338 w1354 w1366 w1376 w1401] -> w1300
              tunnel: w1298 -> [w1317 _ _ _ _ w1396]
              tunnel: [w1314 w1334 w1350 w1361 w1370 w1394] -> w1297
              tunnel: w1294 -> [w1313 w1331 w1347 w1360 w1369 w1391]
              tunnel: w1293 -> [w1312 w1330 w1346 w1359 w1368 w1390]
              tunnel: [w1313 w1331 w1345 w1360 w1369 w1393] -> w1292
              tunnel: [w1312 w1330 w1344 w1359 w1368 w1392] -> w1291
              frame "$R" {
                w1314 = "$V0R" ("write buffer")
                n662 = String Subset(string=w1317, offset (0)=2, length (rest)=2 ("length (rest)")) -> (substring=w1316:string)
                n663 = case shown="\"00\"" w1316 {
                  frame "01" {
                    n664 = property on="RIGHT" class="Bool (strict)"("Value (Signaling)"=TRUE) -> (error out=w1326:errorcluster)  [unwired: 2 in, 1 out]
                    n665 = property on="RIGHT" class="Bool (strict)"(error in=w1326, "Value"=FALSE ("Value (Signaling)")) -> ()  [unwired: 1 in, 2 out]
                  }
                  frame Default {
                  }
                  frame "00" {
                    n666 = property on="WRONG" class="Bool (strict)"("Value (Signaling)"=TRUE) -> (error out=w1329:errorcluster)  [unwired: 2 in, 1 out]
                    n667 = property on="WRONG" class="Bool (strict)"(error in=w1329, "Value"=FALSE ("Value (Signaling)")) -> ()  [unwired: 1 in, 2 out]
                  }
                }
                n668 = property on="Communication" class="Bool (strict)"("Value"=TRUE ("Communication")) -> ()  [unwired: 2 in, 2 out]
                n669 = VISA Write(VISA resource name=w1321, write buffer=w1314, error in (no error)=w1320) -> (VISA resource name out=w1322:refnum<visa-resource-name>, error out=w1323:errorcluster)  [unwired: 1 out]
              }
              frame "$N" {
                w1334 = "$V0N" ("write buffer")
                n670 = property on="Start New Question" class="Bool (strict)"("Value (Signaling)"=TRUE) -> (error out=w1340:errorcluster)  [unwired: 2 in, 1 out]
                n671 = property on="Communication" class="Bool (strict)"("Value"=TRUE ("Communication")) -> ()  [unwired: 2 in, 2 out]
                n672 = property on="Start New Question" class="Bool (strict)"(error in=w1340, "Value"=FALSE ("Value (Signaling)")) -> ()  [unwired: 1 in, 2 out]
                n673 = property on="Team / Player" class="Str"("Value"="" ("Team / Player"), "Blinking"=FALSE) -> ()  [unwired: 2 in, 2 out]
                n674 = VISA Write(VISA resource name=w1337, write buffer=w1334, error in (no error)=w1336) -> (VISA resource name out=w1339:refnum<visa-resource-name>, error out=w1338:errorcluster)  [unwired: 1 out]
              }
              frame "$H" {
                w1350 = "$V0H" ("write buffer")
                n675 = property on="Start New Question" class="Bool (strict)"("Value (Signaling)"=TRUE) -> (error out=w1356:errorcluster)  [unwired: 2 in, 1 out]
                n676 = property on="Communication" class="Bool (strict)"("Value"=TRUE ("Communication")) -> ()  [unwired: 2 in, 2 out]
                n677 = property on="Start New Question" class="Bool (strict)"(error in=w1356, "Value"=FALSE ("Value (Signaling)")) -> ()  [unwired: 1 in, 2 out]
                n678 = property on="Team / Player" class="Str"("Value"="" ("Team / Player"), "Blinking"=FALSE) -> ()  [unwired: 2 in, 2 out]
                n679 = VISA Write(VISA resource name=w1353, write buffer=w1350, error in (no error)=w1352) -> (VISA resource name out=w1355:refnum<visa-resource-name>, error out=w1354:errorcluster)  [unwired: 1 out]
                n680 = Enqueue Element(queue=w1347, element="TIMER0" ("string"), error in (no error)=w1346) -> (queue out=w1345:refnum<queue>, error out=w1344:errorcluster)  [unwired: 1 in, 1 out]
              }
              frame "$U" {
                w1361 = "$V0U" ("write buffer")
                n681 = property on="Timeout" class="Bool (strict)"("Value"=TRUE ("Timeout")) -> ()  [unwired: 2 in, 2 out]
                n682 = property on="Communication" class="Bool (strict)"("Value"=TRUE ("Communication")) -> ()  [unwired: 2 in, 2 out]
                n683 = VISA Write(VISA resource name=w1365, write buffer=w1361, error in (no error)=w1364) -> (VISA resource name out=w1367:refnum<visa-resource-name>, error out=w1366:errorcluster)  [unwired: 1 out]
              }
              frame Default {
                w1370 = "$I00" ("write buffer")
                n684 = Wait (ms)(milliseconds to wait=u32 500) -> ()  [unwired: 1 out]
                n685 = property on="Communication" class="Bool (strict)"("Value"=FALSE ("Communication")) -> ()  [unwired: 2 in, 2 out]
                n686 = VISA Write(VISA resource name=w1374, write buffer=w1370, error in (no error)=w1373) -> (VISA resource name out=w1375:refnum<visa-resource-name>, error out=w1376:errorcluster)  [unwired: 1 out]
              }
              frame "$B" {
                w1394 = "$V0B" ("write buffer")
                n687 = property on="Answer Time" class="DigNum (strict)"() -> ("Value"=w1386:u8)  [unwired: 2 in, 2 out]
                n688 = property on="Communication" class="Bool (strict)"("Value"=TRUE ("Communication")) -> ()  [unwired: 2 in, 2 out]
                n689 = String Subset(string=w1396, offset (0)=2, length (rest)=1 ("length (rest)")) -> (substring=w1384:string)
                n690 = String Subset(string=w1396, offset (0)=3, length (rest)=1 ("length (rest)")) -> (substring=w1382:string)
                n691 = Number To Decimal String(number=w1386) -> (decimal integer string=w1388:string)  [unwired: 1 in]
                n692 = Decimal String To Number(string=w1384) -> (number=w1399:i32)  [unwired: 2 in, 1 out]
                n693 = Decimal String To Number(string=w1382) -> (number=w1395:i32)  [unwired: 2 in, 1 out]
                n694 = Concatenate Strings("BUTTON PRESSED: Team " ("string"), w1384, " Player " ("string"), w1382) -> (w1381:string)
                n695 = property on="Team Pressed" class="DigNum (strict)"("Value"=w1399) -> ()  [unwired: 2 in, 2 out]
                n696 = property on="Button Pressed" class="DigNum (strict)"("Value"=w1395) -> ()  [unwired: 2 in, 2 out]
                n697 = Concatenate Strings("TIMER" ("string"), w1388) -> (w1387:string)
                n698 = flat-sequence {
                  tunnel: [w1407] -> w1379
                  tunnel: w1379 -> [w1408]
                  frame #0 {
                    w1407 = 400.0 ("frequency (Hz) - ignored")
                    n699 = call <vilib>:"Beep.vi"("frequency (Hz)"=w1407) -> ()  [unwired: 11 in]
                  }
                  frame #1 {
                    n700 = call <vilib>:"Beep.vi"("frequency (Hz)"=w1408) -> ()  [unwired: 11 in]
                  }
                }
                n701 = property on="Team / Player" class="Str"("Value"=w1381, "Blinking"=TRUE) -> ()  [unwired: 2 in, 2 out]
                n702 = Enqueue Element(queue=w1391, element=w1387, error in (no error)=w1390) -> (queue out=w1393:refnum<queue>, error out=w1392:errorcluster)  [unwired: 1 in, 1 out]
                n703 = VISA Write(VISA resource name=w1404, write buffer=w1394, error in (no error)=w1403) -> (VISA resource name out=w1402:refnum<visa-resource-name>, error out=w1401:errorcluster)  [unwired: 1 out]
                n704 = property on="WRONG" class="Bool (strict)"("Disabled"=u8 0) -> ()  [unwired: 2 in, 2 out]
                n705 = property on="RIGHT" class="Bool (strict)"("Disabled"=u8 0) -> ()  [unwired: 2 in, 2 out]
              }
            }
            n706 = Concatenate Strings(w1299, w1298, w1297, "\r") -> (w1296:string)
          }
        }
        n707 = property on="Com Msgs" class="Str"("Value"=w1256) -> ()  [unwired: 2 in, 2 out]
      }
      frame Error {
        n708 = property on="COM Port" class="VISAName"() -> ("Value"=w1488:refnum<visa-resource-name>)  [unwired: 2 in, 2 out]
        n709 = VISA Close(VISA resource name=w1488) -> (error out=w1489:errorcluster)  [unwired: 1 in]
        n710 = call-poly "VISA Configure Serial Port"("VISA resource name"=w1488, "timeout (10sec)"=u32 1000, "Enable Termination\nChar (T)"=FALSE ("Enable Termination\nChar (T)"), "baud rate (9600)"=u32 115200, "error in (no error)"=w1489) -> ("VISA resource name out"=w1484:refnum<visa-resource-name>, "error out"=w1483:errorcluster)  [unwired: 9 in]
        n711 = case shown="Error" w1483 {
          frame No Error {
            n712 = property on="COM Port" class="Bool (strict)"("Value"=TRUE ("COM Port")) -> ()  [unwired: 2 in, 2 out]
          }
          frame Error {
            n713 = property on="COM Port" class="Bool (strict)"("Value"=FALSE ("COM Port")) -> ()  [unwired: 2 in, 2 out]
          }
        }
      }
    }
    n714 = property on="stop" class="Bool (strict)"() -> ("Value"=w1249:bool)  [unwired: 2 in, 2 out]
  }
  n715 = Release Queue(queue=w25, error in (no error)=w24) -> (error out=w22:errorcluster)  [unwired: 1 in, 2 out]
  n716 = VISA Close(VISA resource name=w26) -> ()  [unwired: 1 in, 1 out]
  n717 = Release Queue(queue=w13, error in (no error)=w12) -> ()  [unwired: 1 in, 3 out]
  n718 = Merge Errors(w22, w21) -> (w23:errorcluster)
  n719 = call <vilib>:"General Error Handler.vi"("error in (no error)"=w23) -> ()  [unwired: 10 in, 5 out]
  n720 = Release Queue(queue=w58, error in (no error)=w57) -> (error out=w44:errorcluster)  [unwired: 1 in, 2 out]
  n721 = Release Queue(queue=w64, error in (no error)=w63) -> (error out=w43:errorcluster)  [unwired: 1 in, 2 out]
  n722 = Merge Errors(w44, w43) -> (w45:errorcluster)
  n723 = call <vilib>:"General Error Handler.vi"("error in (no error)"=w45) -> ()  [unwired: 10 in, 5 out]
  "Question" <- w4
  "Answer" <- w4
  "GameGUI" <- bool[][] [[FALSE, FALSE, FALSE, FALSE, FALSE, FALSE], [FALSE, FALSE, FALSE, FALSE, FALSE, FALSE], [FALSE, FALSE, FALSE, FALSE, FALSE, FALSE], [FALSE, FALSE, FALSE, FALSE, FALSE, FALSE], [FALSE, FALSE, FALSE, FALSE, FALSE, FALSE]] ("GameGUI")
  "Used 2" <- w4
  "Used 3" <- w4
  "Used 4" <- w4
  "Used 5" <- w4
  "Used 6" <- w4
  "Used 1" <- w4
  "Communication" <- FALSE ("Connected")
  "COM Port" <- FALSE ("COM Port")
  "Timeout" <- FALSE ("Timeout")
  "Com Msgs" <- "" ("Com Msgs")
  "Used 7" <- w4
  "Is Daily Double or Final Jeopardy" <- FALSE ("Is Final Jeopardy")
  "Game Started" <- FALSE ("Game Started")
  "Stats" <- i32[] [0, 0, 0, 0, 0, 0, 0, 0, 0]
